vi "test.vi"() -> ()   [LabVIEW 2019]
uses:
  <vilib>/Math Plots/3D Math Plots/3D Surface/3D Surface XCtrl/3D Surface.xctl
  <vilib>/Math Plots/3D Math Plots/3D Surface/3D Surface Datatype/Public/Plot Helper (Vector).vi
  <vilib>/Analysis/NI_AALBase.lvlib
  <vilib>/Math Plots/3D Math Plots/3D Surface/3D Surface Datatype/3D Surface Datatype.lvclass
panel:
  out "appended array":u32[][](array[numeric])
  out "output array":i32[][](array[numeric])
  out "CZT Count Map":refnum<class "3D Plot Datatype.lvclass">[](xcontrol)
  out "Histogram Graph":T1(graph)
  out "Channel":u32[](array[numeric])
  out "Energy":u32[](array[numeric])
  out "Chan+Energy":u32[](array[numeric]) format="%.0x"
  out "Clk Ticks":u32[](array[numeric])
  out "Sr No":i32[](array[numeric])
  # "Sr. No."
  # "Clk Tick"
  # "Raw Data"
  # "Channel"
  # "Energy"
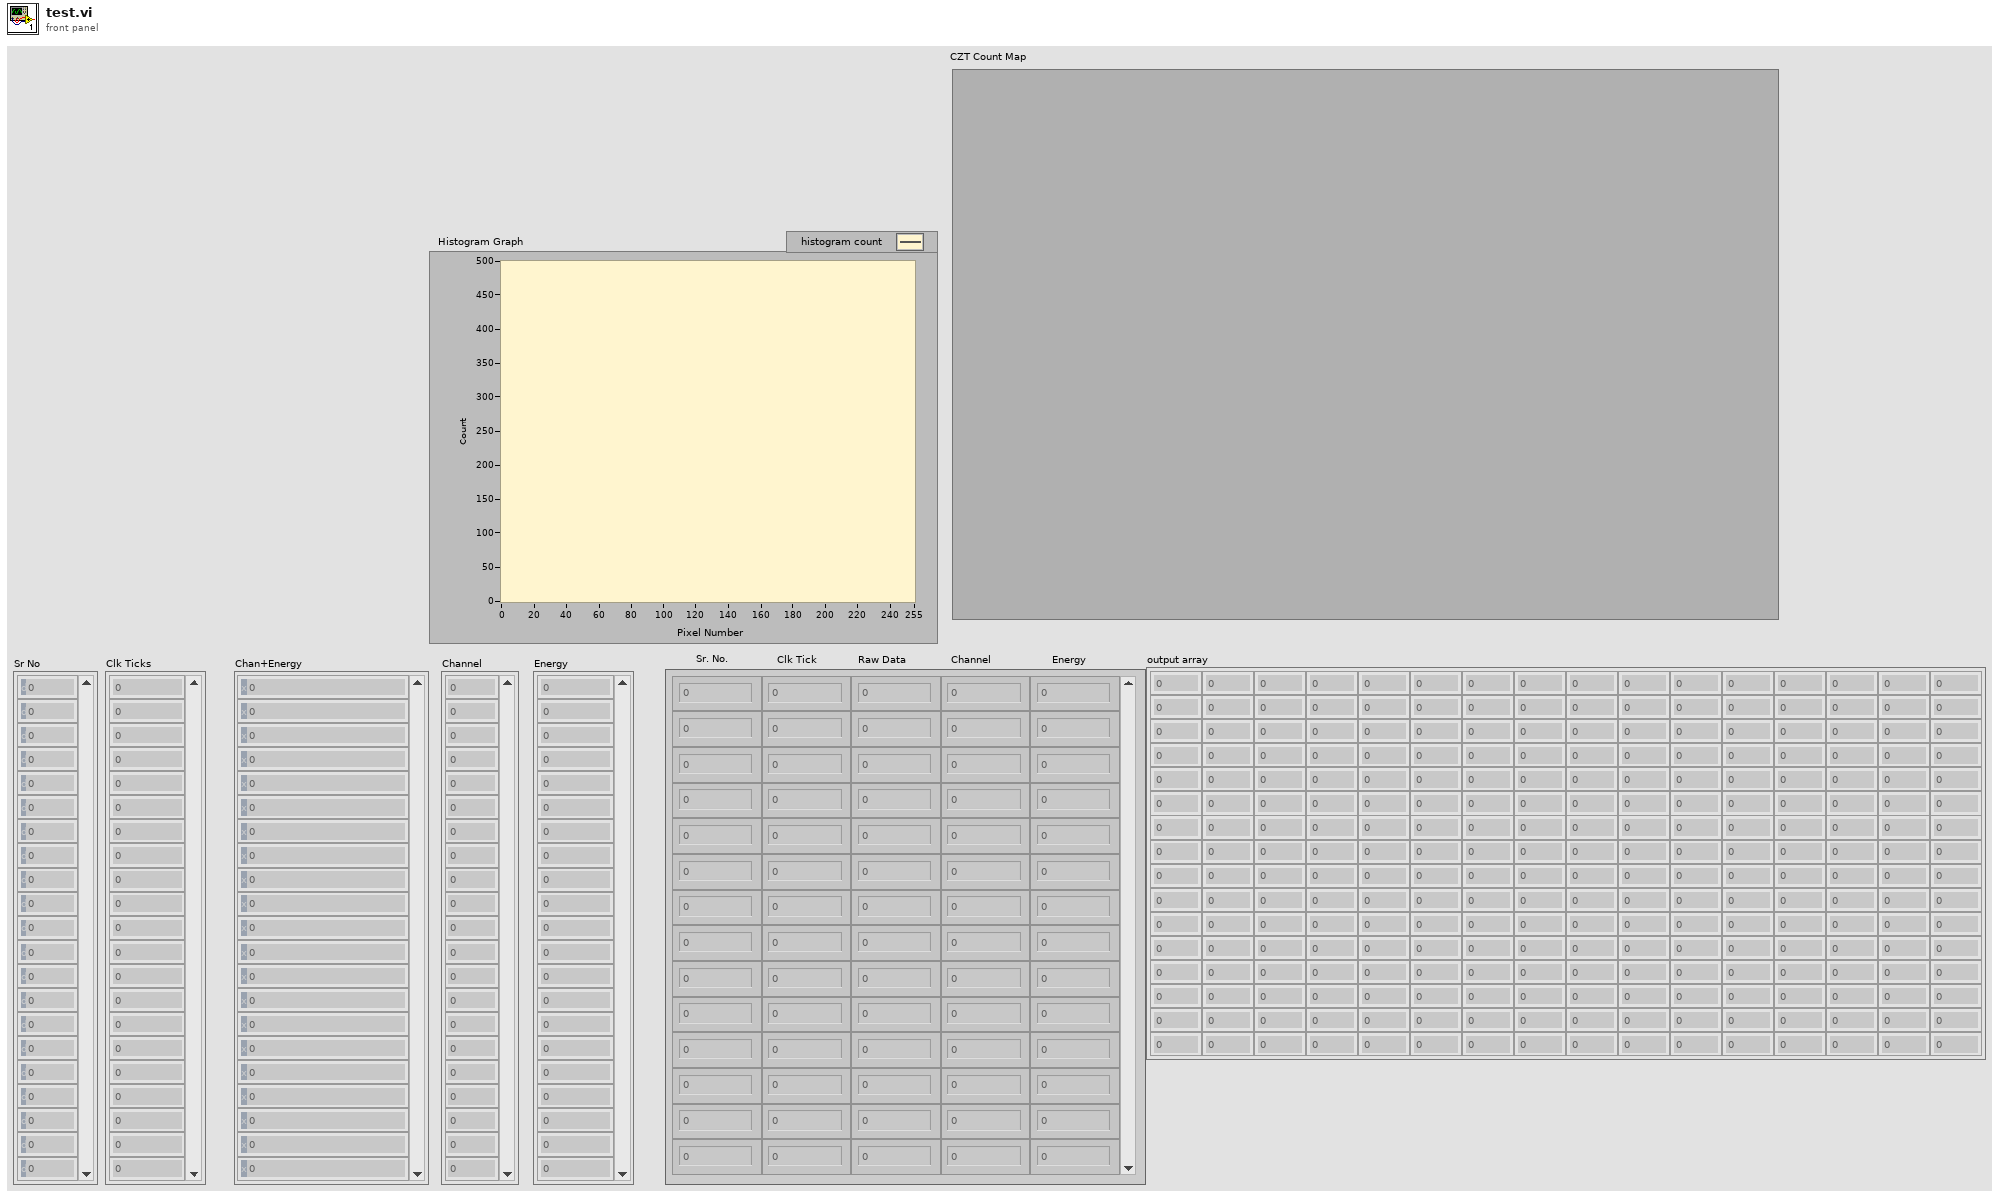
[diagram p1: front panel]
types:
  T1 = cluster{"X Values":dbl[], "Histogram: h(x)":i32[]}
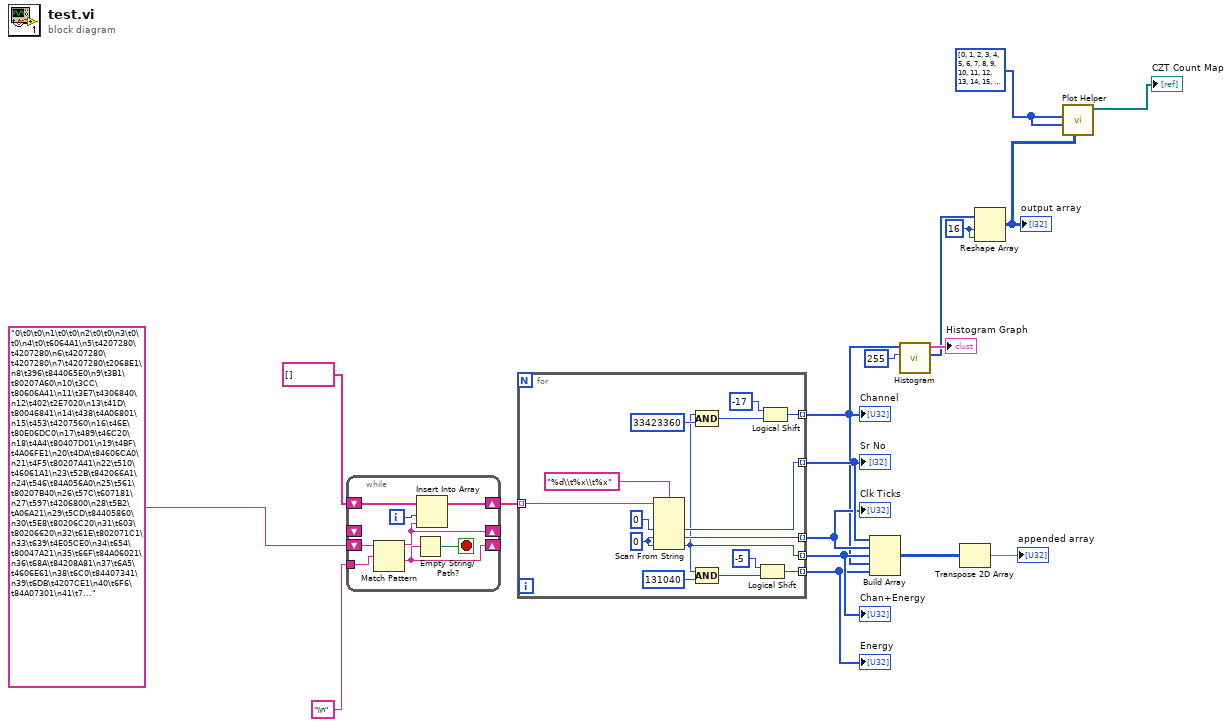
[diagram p0: block diagram]
diagram:
  w1 = u8[] [0, 1, 2, 3, 4, 5, 6, 7, 8, 9, 10, 11, 12, 13, 14, 15, 0, 1, 2, 3, 4, 5, 6, 7, 8, 9, 10, 11, 12, 13, 14, 15, 0, 1, 2, 3, 4, 5, 6, 7, 8, 9, 10, 11, 12, 13, 14, 15, 0, 1, 2, 3, 4, 5, 6, 7, 8, 9, 10, 11, 12, 13, 14, 15, 0, 1, 2, 3, 4, 5, 6, 7, 8, 9, 10, 11, 12, 13, 14, 15, 0, 1, 2, 3, 4, 5, 6, 7, 8, 9, 10, 11, 12, 13, 14, 15, 0, 1, 2, 3, 4, 5, 6, 7, 8, 9, 10, 11, 12, 13, 14, 15, 0, 1, 2, 3, 4, 5, 6, 7, 8, 9, 10, 11, 12, 13, 14, 15, 0, 1, 2, 3, 4, 5, 6, 7, 8, 9, 10, 11, 12, 13, 14, 15, 0, 1, 2, 3, 4, 5, 6, 7, 8, 9, 10, 11, 12, 13, 14, 15, 0, 1, 2, 3, 4, 5, 6, 7, 8, 9, 10, 11, 12, 13, 14, 15, 0, 1, 2, 3, 4, 5, 6, 7, 8, 9, 10, 11, 12, 13, 14, 15, 0, 1, 2, 3, 4, 5, 6, 7, 8, 9, 10, 11, 12, 13, 14, 15, 0, 1, 2, 3, 4, 5, 6, 7, 8, 9, 10, 11, 12, 13, 14, 15, 0, 1, 2, 3, 4, 5, 6, 7, 8, 9, 10, 11, 12, 13, 14, 15, 0, 1, 2, 3, 4, 5, 6, 7, 8, 9, 10, 11, 12, 13, 14] ("Array")
  w4 = 16
  n1 = while {
    tunnel: "\\n" ("regular expression") -> [w25]
    shift-right: [w23] -> _
    shift-left: _ -> [_]
    shift-right: [w20] -> _
    shift-left: "0\t0\t0\n1\t0\t0\n2\t0\t0\n3\t0\t0\n4\t0\t6064A1\n5\t4207280\t4207280\n6\t4207280\t4207280\n7\t4207280\t2068E1\n8\t396\t844065E0\n9\t3B1\t80207A60\n10\t3CC\t80606A41\n11\t3E7\t4306840\n12\t402\t2E7020\n13\t41D\t80046841\n14\t438\t4A06801\n15\t453\t4207560\n16\t46E\t80E06DC0\n17\t489\t46C20\n18\t4A4\t80407D01\n19\t4BF\t4A06FE1\n20\t4DA\t84606CA0\n21\t4F5\t80207A41\n22\t510\t46061A1\n23\t52B\t842066A1\n24\t546\t84A056A0\n25\t561\t80207B40\n26\t57C\t607181\n27\t597\t4206800\n28\t5B2\tA06A21\n29\t5CD\t84405860\n30\t5E8\t80206C20\n31\t603\t80206620\n32\t61E\t802071C1\n33\t639\t4E05CE0\n34\t654\t80047A21\n35\t66F\t84A06021\n36\t68A\t84208A81\n37\t6A5\t4606E61\n38\t6C0\t84407341\n39\t6DB\t4207CE1\n40\t6F6\t84A07301\n41\t711\t4606C60\n42\t72C\t80406D00\n43\t747\t207EE0\n44\t762\t802070A0\n45\t77D\t80406620\n46\t798\t80208AC0\n47\t7B3\t607481\n48\t7CE\t4208900\n49\t7E9\t3871C1\n50\t804\t42E7E21\n51\t81F\t85706541\n52\t83A\t4E06A61\n53\t855\t84506DE0\n54\t870\t80047AA0\n55\t88B\t80307601\n56\t8A6\t4A07C80\n57\t8C1\t20A361\n58\t8DC\t844084E0\n59\t8F7\t80206C80\n60\t912\t6083A1\n61\t92D\t842071A1\n62\t948\t844078A1\n63\t963\t84606AA0\n64\t97E\t80206160\n65\t999\t80206E21\n66\t9B4\t84E05D00\n67\t9CF\t470A0\n68\t9EA\t80A06921\n69\tA05\t84208021\n70\tA20\t84407840\n71\tA3B\t606CE1\n72\tA56\t842067A0\n73\tA71\t80206F40\n74\tA8C\t2075E1\n75\tAA7\t84206920\n76\tAC2\t80206B81\n77\tADD\t44074C1\n78\tAF8\t4047840\n79\tB13\t1846AC1\n80\tB2E\t46061E0\n81\tB49\t80208321\n82\tB64\t84406E60\n83\tB7F\t80206F01\n84\tB9A\t4206920\n85\tBB5\t80206661\n86\tBD0\t84207A60\n87\tBEB\t80608040\n88\tC06\t208381\n89\tC21\t4406B00\n90\tC3C\t206DA0\n91\tC57\t80206860\n92\tC72\t80206A80\n93\tC8D\t206CE0\n94\tCA8\t80206141\n95\tCC3\t4406561\n96\tCDE\t84207D61\n97\tCF9\t84207CE1\n98\tD14\t84306D61\n99\tD2F\t84E065C1\n100\tD4A\t4047120\n101\tD65\t80A067C1\n102\tD80\t4208D80\n103\tD9B\t607D00\n104\tDB6\t408220\n105\tDD1\t80208E01\n106\tDEC\t4605E80\n107\tE07\t406AA1\n108\tE22\t842071A1\n109\tE3D\t84207660\n110\tE58\t80206BE1\n111\tE73\t842061C0\n112\tE8E\t206540\n113\tEA9\t206EA0\n114\tEC4\t80206181\n115\tEDF\t42069C1\n116\tEFA\t4406F20\n117\tF15\t80207240\n118\tF30\t207021\n119\tF4B\t84406400\n120\tF66\t208321\n121\tF81\t84207880\n122\tF9C\t2077A1\n123\tFB7\t84206C40\n124\tFD2\t605EE0\n125\tFED\t800468E1\n126\t1008\t84406B81\n127\t1023\t42090A1\n128\t103E\t842072C1\n129\t1059\t4FC5921\n130\t1074\t85AE7421\n131\t108F\t84F073C1\n132\t10AA\t5C268E0\n133\t10C5\t80387021\n134\t10E0\t850E6C21\n135\t10FB\t84327E61\n136\t1116\t84E08EA1\n137\t1131\t859075C0\n138\t114C\t12E5620\n139\t1167\t80D07581\n140\t1182\t4048861\n141\t119D\t85507041\n142\t11B8\t42E83A1\n143\t11D3\t84707060\n144\t11EE\t80A08F61\n145\t1209\t85706081\n146\t1224\t44E6EA1\n147\t123F\t84B06181\n148\t125A\t420B981\n149\t1275\t4307A61\n150\t1290\t848E70E0\n151\t12AB\t80906F00\n152\t12C6\t6092A1\n153\t12E1\t84365F00\n154\t12FC\t409061\n155\t1317\t84507F61\n156\t1332\t84206301\n157\t134D\t4205A01\n158\t1368\t4A05220\n159\t1383\t80046700\n160\t139E\t607A20\n161\t13B9\t80207740\n162\t13D4\t4077C1\n163\t13EF\t40458E1\n164\t140A\t84606CE1\n165\t1425\t84208440\n166\t1440\t4065E0\n167\t145B\t80305480\n168\t1476\t2E8520\n169\t1491\t80366740\n170\t14AC\t47BC1\n171\t14C7\t4507CA1\n172\t14E2\t84E07000\n173\t14FD\t20A680\n174\t1518\tA08200\n175\t1533\t607841\n176\t154E\t4409160\n177\t1569\t80205B41\n178\t1584\t4205F20\n179\t159F\t81DC52C1\n180\t15BA\t58E7500\n181\t15D5\t1D275A0\n182\t15F0\t81C66340\n183\t160B\t5C7E60\n184\t1626\t80EE66C0\n185\t1641\t3479A0\n186\t165C\t80E090E0\n187\t1677\t81DC5740\n188\t1692\t16E9321\n189\t16AD\t85307201\n190\t16C8\t5A46921\n191\t16E3\t84388681\n192\t16FE\t42C64E1\n193\t1719\t84D08D80\n194\t1734\t4A2A0\n195\t174F\t81D85EE1\n196\t176A\t85AE9381\n197\t1785\t5D084A0\n198\t17A0\t81C66940\n199\t17BB\t7A72E0\n200\t17D6\t806E6061\n201\t17F1\t84327F00\n202\t180C\tA08C40\n203\t1827\t1DA60E1\n204\t1842\t852E6BE1\n205\t185D\t85B07FC1\n206\t1878\t5C47A61\n207\t1893\t84388261\n208\t18AE\t84286261\n209\t18C9\t843085E0\n210\t18E4\t8020AE21\n211\t18FF\t85DC8001\n212\t191A\t58E7720\n213\t1935\t81D467A0\n214\t1950\t81C290C0\n215\t196B\tBA6601\n216\t1986\t4CE64C0\n217\t19A1\t347A21\n218\t19BC\t84E09A80\n219\t19D7\t5A7121\n220\t19F2\t854E77C1\n221\t1A0D\t51070A1\n222\t1A28\t85A26E01\n223\t1A43\t43A6681\n224\t1A5E\t42C6561\n225\t1A79\t84B06E00\n226\t1A94\t48DA1\n227\t1AAF\t84FC7DE1\n228\t1ACA\t85AE7121\n229\t1AE5\t85D068C1\n230\t1B00\t4327560\n231\t1B1B\t810E6840\n232\t1B36\t3CB200\n233\t1B51\tE079A0\n234\t1B6C\t81D08B60\n235\t1B87\t816E7760\n236\t1BA2\t803C9560\n237\t1BBD\t81C273C1\n238\t1BD8\t4B069A1\n239\t1BF3\t842E6E40\n240\t1C0E\t3C91C1\n241\t1C29\t40460A1\n242\t1C44\t85306E00\n243\t1C5F\t1C860C0\n244\t1C7A\t3CACC0\n245\t1C95\tA07961\n246\t1CB0\t847067E1\n247\t1CCB\t852E6D81\n248\t1CE6\t43C9660\n249\t1D01\t80207900\n250\t1D1C\t1D08700\n251\t1D37\t1AE6E80\n252\t1D52\t3CEDC0\n253\t1D6D\tE07120\n254\t1D88\t80D07000\n255\t1DA3\t12E6920\n256\t1DBE\t803CE760\n257\t1DD9\t80045E00\n258\t1DF4\t19083C0\n259\t1E0F\t406721\n260\t1E2A\t843CB4A0\n261\t1E45\t802089E1\n262\t1E60\t84307181\n263\t1E7B\t4A07C40\n264\t1E96\t3C7501\n265\t1EB1\t42E7AE0\n266\t1ECC\t81D06A21\n267\t1EE7\t84044D01\n268\t1F02\t43CBCA1\n269\t1F1D\t858E6B41\n270\t1F38\t4326D41\n271\t1F53\t4E08EC1\n272\t1F6E\t43C76E0\n273\t1F89\t80209281\n274\t1FA4\t4967601\n275\t1FBF\t48E7460\n276\t1FDA\t80987621\n277\t1FF5\t85C67B01\n278\t2010\t4907301\n279\t202B\t54E82A1\n280\t2046\t851C60E1\n281\t2061\t84606DE0\n282\t207C\t81D480E1\n283\t2097\t842C7861\n284\t20B2\t855C7461\n285\t20CD\t85626F60\n286\t20E8\t80526F20\n287\t2103\t81C88C20\n288\t211E\t80DC6200\n289\t2139\t247221\n290\t2154\t855079C0\n291\t216F\tCE7C41\n292\t218A\t53C7A21\n293\t21A5\t85C46621\n294\t21C0\t843662C1\n295\t21DB\t52E7BC1\n296\t21F6\t4386B21\n297\t2211\t84E0C100\n298\t222C\t1526381\n299\t2247\t4286FA0\n300\t2262\t81BC6B20\n301\t227D\t81847A81\n302\t2298\t4347C21\n303\t22B3\t858E9C61\n304\t22CE\t847C6C01\n305\t22E9\t42677C1\n306\t2304\t5306F61\n307\t231F\t846E73E1\n308\t233A\t84787460\n309\t2355\t81C27340\n310\t2370\tD098A0\n311\t238B\t816E7F80\n312\t23A6\t386721\n313\t23C1\t84A08A80\n314\t23DC\t1D27401\n315\t23F7\t42A61E1\n316\t2412\t85D87E20\n317\t242D\t81026401\n318\t2448\t432A1A0\n319\t2463\t81AE9120\n320\t247E\t80BC6F80\n321\t2499\t4A340\n322\t24B4\t1B07121\n323\t24CF\t84EE7A61\n324\t24EA\t85DCA740\n325\t2505\t1C25960\n326\t2520\t80307CE0\n327\t253B\t818E6121\n328\t2556\t84386C61\n329\t2571\t84E086C0\n330\t258C\t1D67481\n331\t25A7\t42E93C0\n332\t25C2\t17C7400\n333\t25DD\t1A45B80\n334\t25F8\tB08B61\n335\t2613\t84AE7621\n336\t262E\t843C7F80\n337\t2649\t2087E0\n338\t2664\t80B65DA0\n339\t267F\t810E82C0\n340\t269A\t1DA8100\n341\t26B5\t4075E1\n342\t26D0\t84707D20\n343\t26EB\t804E7E41\n344\t2706\t49C7281\n345\t2721\t4047560\n346\t273C\t81926AC0\n347\t2757\tA08841\n348\t2772\t43A7241\n349\t278D\t4207161\n350\t27A8\t849084E1\n351\t27C3\t84E06580\n352\t27DE\t5A8741\n353\t27F9\t4047761\n354\t2814\t857063C0\n355\t282F\t607721\n356\t284A\t843C76C1\n357\t2865\t5AE7421\n358\t2880\t84327300\n359\t289B\t1C26861\n360\t28B6\t85DC65E1\n361\t28D1\t842E8080\n362\t28EC\t1D07E00\n363\t2907\t20BAC0\n364\t2922\t7A76E1\n365\t293D\t858E6160\n366\t2958\t80307A20\n367\t2973\t80E086C0\n368\t298E\t5C7CA1\n369\t29A9\t850E6A21\n370\t29C4\t851069E1\n371\t29DF\t840497E1\n372\t29FA\t84FC7221\n373\t2A15\t84A06D80\n374\t2A30\tD07560\n375\t2A4B\t80205FA1\n376\t2A66\t843C74A0\n377\t2A81\t80E06D41\n378\t2A9C\t5D07481\n379\t2AB7\t56E7020\n380\t2AD2\t81DC6280\n381\t2AED\t1C26E80\n382\t2B08\t327DC1\n383\t2B23\t42E72A0\n384\t2B3E\t80387EA1\n385\t2B59\t840491E1\n386\t2B74\t85907BE0\n387\t2B8F\t81AE7B00\n388\t2BAA\tFC5FC0\n389\t2BC5\t406A80\n390\t2BE0\t508040\n391\t2BFB\t4E5840\n392\t2C16\t3C88E1\n393\t2C31\t8420A320\n394\t2C4C\t80F07E21\n395\t2C67\t858E7360\n396\t2C82\t80B05F01\n397\t2C9D\t4E08180\n398\t2CB8\t15070A0\n399\t2CD3\t80CE6020\n400\t2CEE\t80309581\n401\t2D09\t4206FC1\n402\t2D24\t5B06D40\n403\t2D3F\tA08FC1\n404\t2D5A\t4905DC1\n405\t2D75\t46096C0\n406\t2D90\t1707181\n407\t2DAB\t44061A0\n408\t2DC6\t80707F41\n409\t2DE1\t4046580\n410\t2DFC\t306C60\n411\t2E17\t80E070A0\n412\t2E32\t80208261\n413\t2E4D\t84A07F20\n414\t2E68\t80206221\n415\t2E83\t84607400\n416\t2E9E\t407740\n417\t2EB9\t2063C1\n418\t2ED4\t4205E00\n419\t2EEF\t1D05A21\n420\t2F0A\t85AE7901\n421\t2F25\t4327220\n422\t2F40\t80E07000\n423\t2F5B\tF07361\n424\t2F76\t842E6701\n425\t2F91\t4386DA0\n426\t2FAC\t81C27A20\n427\t2FC7\t80365D01\n428\t2FE2\t58E6BA0\n429\t2FFD\t81D069E1\n430\t3018\t84047DE0\n431\t3033\t80328120\n432\t304E\t802E6820\n433\t3069\t81B06E61\n434\t3084\t84A087A0\n435\t309F\t80306060\n436\t30BA\t81AE75E0\n437\t30D5\t80707740\n438\t30F0\t208AC0\n439\t310B\t507C01\n440\t3126\t4E07581\n441\t3141\t4608FE0\n442\t315C\t80408AC0\n443\t3177\t205D21\n444\t3192\t84205AC1\n445\t31AD\t4605B01\n446\t31C8\t4047461\n447\t31E3\t84406920\n448\t31FE\t802080A0\n449\t3219\t80205E00\n450\t3234\tA05FC0\n451\t324F\t471C1\n452\t326A\t4607400\n453\t3285\t2076A0\n454\t32A0\t804071E0\n455\t32BB\t802070E1\n456\t32D6\t85D85D21\n457\t32F1\t848E7DC0\n458\t330C\t1D474C1\n459\t3327\t5C66141\n460\t3342\t45A7340\n461\t335D\t12E6680\n462\t3378\t328341\n463\t3393\t4E09160\n464\t33AE\t81DA62A1\n465\t33C9\t842C6E00\n466\t33E4\t1306061\n467\t33FF\t1A46541\n468\t341E\t388E40\n469\t3451\t18E6C01\n470\t3482\tD08541\n471\t34B5\t493E0\n472\t34E6\t1DC6341\n473\t3519\tEE7160\n474\t354A\t1D07800\n475\t357D\t1C265E1\n476\t35AE\t3C7FC1\n477\t35E1\t14E5B00\n478\t3612\t3085E0\n479\t3645\tA09120\n480\t3676\tFC67E0\n481\t36A9\t2E8B60\n482\t36DA\t15063E0\n483\t370D\t20B401\n484\t373E\tB06881\n485\t3771\t1AE6E20\n486\t37A2\t1D879A0\n487\t37D5\t1C65D81\n488\t3806\t1D26800\n489\t3839\t6E7581\n490\t386A\t3863E0\n491\t389D\tE06E60\n492\t38CE\t327401\n493\t3901\t16E6660\n494\t3932\t1DC7601\n495\t3965\t1A46101\n496\t3996\t1107361\n497\t39C9\t2E85A1\n498\t39FA\t3C6820\n499\t3A2D\t46821\n500\t3A5E\t707FC0\n501\t3A91\t18E6F20\n502\t3AC2\t1DC7FC1\n503\t3AF5\t1C45D80\n504\t3B26\t1D08121\n505\t3B59\tCE6F80\n506\t3B8A\t325FC1\n507\t3BBD\t60A600\n508\t3BEE\t19067A0\n509\t3C21\t1AE7721\n510\t3C52\tD07A21\n511\t3C85\t1C26000\n512\t3CB6\t3877C1\n513\t3CE9\t2E8301\n514\t3D1A\t1D26400\n515\t3D4D\t207021\n516\t3D7E\t1DC6A81\n517\t3DB1\t12E6BC0\n518\t3DE2\t326F61\n519\t3E15\tE081A1\n520\t3E46\t3A6E80\n521\t3E79\tAE62E1\n522\t3EAA\t13067C0\n523\t3EDD\t46D21\n524\t3F0E\t385241\n525\t3F41\t18E7921\n526\t3F72\t308281\n527\t3FA5\t1C27241\n528\t3FD6\t3C8E21\n529\t4009\t2E74A0\n530\t403A\t1D06AE1\n531\t406D\tA07C20\n532\t409E\t327941\n533\t40D1\t16E7301\n534\t4102\t1D85EA0\n535\t4135\t1C475E0\n536\t4166\t1706EA1\n537\t4199\t10E60C0\n538\t41CA\t388780\n539\t41FD\t208681\n540\t422E\t906880\n541\t4261\t1C88561\n542\t4292\t1BC6220\n543\t42C5\t1C67761\n544\t42F6\t1B26F20\n545\t4329\t2A6821\n546\t435A\tBC6640\n547\t438D\tE08041\n548\t43BE\t526421\n549\t43F1\tEC6F20\n550\t4422\t17C6DC1\n551\t4455\t1426FE0\n552\t4486\tF07800\n553\t44B9\t4E7721\n554\t44EA\t11C73E0\n555\t451D\t48321\n556\t454E\t367760\n557\t4581\t18E67C0\n558\t45B2\t1DC75C1\n559\t45E5\t1C27B60\n560\t4616\t1D66120\n561\t4649\t287AC1\n562\t467A\t7C6AC1\n563\t46AD\t409601\n564\t46DE\t3482A1\n565\t4711\t14E65C1\n566\t4742\t1D881E0\n567\t4775\t1026861\n568\t47A6\t1B06CE1\n569\t47D9\tCE7BA1\n570\t480A\t3872C1\n571\t483D\t206400\n572\t486E\tD07A41\n573\t48A1\t1AE52A1\n574\t48D2\t1DA8741\n575\t4905\t1825E60\n576\t4936\t1D45C61\n577\t4969\t2C78E0\n578\t499A\t5A6FE1\n579\t49CD\tA066A0\n580\t49FE\t327801\n581\t4A31\t12E8801\n582\t4A62\t3C6740\n583\t4A95\t1A46921\n584\t4AC6\t1307861\n585\t4AF9\t8E7421\n586\t4B2A\tFC72E1\n587\t4B5D\t207420\n588\t4B8E\t306780\n589\t4BC1\t16E6960\n590\t4BF2\t5C84E1\n591\t4C25\t1A26000\n592\t4C56\t1D06C00\n593\t4C89\t2E6B61\n594\t4CBA\t3A7700\n595\t4CED\tE06B81\n596\t4D1E\tB06700\n597\t4D51\tEE6DE0\n598\t4D82\t1506680\n599\t4DB5\t1C46381\n600\t4DE6\t7082C1\n601\t4E19\t6E6DE1\n602\t4E4A\t1D27EC1\n603\t4E7D\t2081A1\n604\t4EAE\t507AE0\n605\t4EE1\t10E9060\n606\t4F12\t1106581\n607\t4F45\t608AE0\n608\t4F76\t1907161\n609\t4FA9\tAE6DA0\n610\t4FDA\t1708080\n611\t500D\t207A60\n612\t503E\t405E41\n613\t5071\t606EE0\n614\t50A2\t206AA1\n615\t50EF\t607061\n616\t5120\t205F40\n617\t5E99\t206441\n618\t835E\t206B00\n619\t88DB\t205580\n620\t8AAC\tE05940\n621\t93B7\t2091A0\n622\t93E8\tA06E40\n623\t941B\t406AC1\n624\t944C\t6072A0\n625\t947F\t206580\n626\tB314\t206540\n627\tB457\t205E81\n628\tB80E\t2063C1\n629\tD0F7\t207261\n630\tE6C2\t606941\n631\tE7ED\t206BE1\n632\tE81E\t206C61\n633\tEDC1\t207681\n634\tEF78\t2066E0\n635\tF0A3\t207300\n636\tF5EA\t207521\n637\tF679\t2073C0\n638\tF88C\t206421\n639\tF969\t2073E1\n640\tF9F6\t606900\n641\tFB6F\t2070E1\n642\tFBA0\t606EA1\n643\tFBD3\t2073A0\n644\tFC04\t206E00\n645\tFD77\t206DE1\n646\tFEA2\t206EA0\n647\tFEEF\t206EA0\n648\tFF3E\tA05D40\n649\tFFCD\t476E1\n650\tFFFE\t407360\n651\t10031\t2083C0\n652\t10062\t606F60\n653\t10095\t205CE0\n654\t10134\tD06181\n655\t103E9\t2E71A0\n656\t1041A\t3072C0\n657\t1044D\tE06A61\n658\t1047E\t506140\n659\t104B1\t47D61\n660\t104E2\tA077E1\n661\t10515\t20A361\n662\t10546\t407A21\n663\t10579\t6078E1\n664\t105AA\t206920\n665\t10769\t4070C0\n666\t107F6\t47081\n667\t10829\t607741\n668\t1085A\t208880\n669\t1088D\t206160\n670\t108E0\t208000\n671\t10923\t2066C1\n672\t10D3C\tD06C01\n673\t110BD\t2E6B20\n674\t110EE\tE06DC0\n675\t11121\t46E81\n676\t11152\tA06180\n677\t11185\t2082E0\n678\t111B6\t406901\n679\t111E9\t606DA1\n680\t1121A\t206080\n681\t1126F\t208720\n682\t11432\t207140\n683\t11721\t4074C1\n684\t117B2\t208041\n685\t117E5\t606F21\n686\t11816\t326F20\n687\t11977\t2E7400\n688\t119A8\t7A6FE0\n689\t119DB\t1C263A0\n690\t11A0C\t3074E1\n691\t11A3F\t48A60\n692\t11A70\tD07280\n693\t11AA3\tE08240\n694\t11AD4\t706F20\n695\t11B07\t20AB00\n696\t11B38\t5071A0\n697\t11B6B\tA08020\n698\t11B9C\t409700\n699\t11BCF\t608301\n700\t11C00\t1D863A1\n701\t11CF7\t12E70E1\n702\t11D28\t13068A0\n703\t11D5B\t1C65AA1\n704\t11D8C\t387000\n705\t11DBF\tCE6940\n706\t11DF0\t327AC0\n707\t11E23\t49CE0\n708\t11E54\t1506C20\n709\t11E87\t16E5140\n710\t11EB8\t906F00\n711\t11EEB\t1A46321\n712\t11F1C\tF08141\n713\t11F4F\t2A5C40\n714\t11F80\t307F40\n715\t11FB3\tE08880\n716\t11FE4\t1706E20\n717\t12017\t4E6F00\n718\t12048\tD07C81\n719\t1207B\t1C26EA1\n720\t120AC\t1107400\n721\t120DF\t2E7A20\n722\t12110\t707F00\n723\t12143\t20AC61\n724\t12174\t366E20\n725\t121A7\tEE6541\n726\t121D8\t508340\n727\t1220B\tA08F20\n728\t1223C\t3072C0\n729\t1226F\t2E71A0\n730\t122A0\t5068A1\n731\t122D3\t485C0\n732\t12304\t8E6E80\n733\t12337\tE08140\n734\t12368\t10E74E1\n735\t1239B\t20A6E0\n736\t123CC\t6E61E1\n737\t123FF\t4091C0\n738\t12430\t609880\n739\t12463\t5A5F00\n740\t125BC\t16E7620\n741\t125EF\t1906821\n742\t12620\t1C27141\n743\t12653\t386D60\n744\t12684\t2E85A1\n745\t126B7\t327CA0\n746\t126E8\t49860\n747\t1271B\tFC6E80\n748\t1274C\tEE4B81\n749\t1277F\t1106CA0\n750\t127B0\tE08360\n751\t127E3\t908020\n752\t12814\t4E7301\n753\t12847\t1506BE1\n754\t12878\t20AB41\n755\t128AB\t308200\n756\t128DC\t10E6B20\n757\t1290F\t17066C0\n758\t12940\tA080C1\n759\t12973\t707480\n760\t129A4\t206821\n761\t129D7\t3673A1\n762\t12A08\t409020\n763\t12A3B\t507E21\n764\t12A6C\t6086A1\n765\t12A9F\t47840\n766\t12AF4\t1846B60\n767\t12B27\tE07120\n768\t12B58\t208581\n769\t12B8B\tA06401\n770\t12BBC\t407DE0\n771\t12BEF\t607200\n772\t12C20\t206E81\n773\t12D4B\t405AC1\n774\t12E74\tF06A81\n775\t12EA7\t470C0\n776\t12ED8\t326361\n777\t12F0B\tE06760\n778\t12F3C\tD07500\n779\t12F6F\t207C21\n780\t12FA0\t306BC1\n781\t12FD3\tA06F81\n782\t13004\t365880\n783\t13037\t206E21\n784\t13068\t506E20\n785\t1309B\tE070C0\n786\t130CC\t6072A0\n787\t130FF\tA060A0\n788\t13130\t405881\n789\t13163\t46781\n790\t133BA\t3276E1\n791\t133ED\t2E6840\n792\t1341E\t906621\n793\t13451\t1846481\n794\t13482\t308580\n795\t134B5\t4E6AE1\n796\t134E6\t366D40\n797\t13519\tE061E1\n798\t1354A\t506440\n799\t1357D\t2E6581\n800\t135AE\t3A6D01\n801\t135E1\t20AAA1\n802\t13612\t306C60\n803\t13645\tA05EA1\n804\t13676\t472E0\n805\t136A9\tE07521\n806\t136DA\t2073A0\n807\t1370D\t607CC1\n808\t1373E\t463E0\n809\t13771\tE068A0\n810\t137A2\t207C81\n811\t137D5\tA06C00\n812\t13806\t477A1\n813\t13839\tE070C0\n814\t1386A\t4069A1\n815\t1389D\t607141\n816\t138CE\t206841\n817\t13901\t406F01\n818\t13932\t205F20\n819\t1398F\t605440\n820\t13AE0\t207401\n821\t13B13\t207740\n822\t13C9E\t2071A1\n823\t13D0F\tF06621\n824\t13E3A\t2E73C1\n825\t13E6D\tD062A0\n826\t13E9E\tE067E1\n827\t13ED1\t506521\n828\t13F02\t47240\n829\t13F35\t307241\n830\t13F66\tA076C1\n831\t13F99\t2092A0\n832\t13FCA\t4084C1\n833\t13FFD\t13C6EA0\n834\t1402E\t1AE8E41\n835\t14061\t1526C41\n836\t14092\t1C673A0\n837\t140C5\t11C6B80\n838\t140F6\tCE6CC1\n839\t14129\tD47460\n840\t1415A\t426EA1\n841\t1418D\t19C7300\n842\t141BE\t12E6601\n843\t141F1\t1B66F41\n844\t14222\t1826961\n845\t14255\tDC7381\n846\t14286\t2C7641\n847\t142B9\tB07401\n848\t142EA\tE09501\n849\t1431D\t17C7181\n850\t1434E\t14E6281\n851\t14381\t1308480\n852\t143B2\t1225F01\n853\t143E5\t387E40\n854\t14416\tAE7600\n855\t14449\t328960\n856\t1447A\t266961\n857\t144AD\t1BC7380\n858\t144DE\t16E84C0\n859\t14511\t15076E1\n860\t14542\t1C28920\n861\t14575\t7C7021\n862\t145A6\t2866C0\n863\t145D9\t708E20\n864\t1460A\tA0A2E0\n865\t1463D\t1D87BA1\n866\t1466E\tEE7B81\n867\t146A1\t966F21\n868\t146D2\t1026D20\n869\t14705\tBC71A1\n870\t14736\t2A6421\n871\t14769\t5274A1\n872\t1479A\t49E81\n873\t147CD\t1DA7C20\n874\t147FE\t6E79E1\n875\t14831\t1907840\n876\t14862\t1A27361\n877\t14895\t5C77C0\n878\t148C6\t2E9480\n879\t148F9\tD071A1\n880\t1492A\tE05980\n881\t1495D\t9C6660\n882\t1498E\t10E7501\n883\t149C1\tF082C0\n884\t149F2\t1A47221\n885\t14A25\t3A68A1\n886\t14A56\t8E7721\n887\t14A89\t3095C0\n888\t14ABA\t20C441\n889\t14AED\t5A7B00\n890\t14B1E\t4E76C1\n891\t14B51\t1708200\n892\t14B82\t1C46CA0\n893\t14BB5\tFC7700\n894\t14BE6\t606D01\n895\t14C19\t908601\n896\t14C4A\t47861\n897\t14C7D\t11084E1\n898\t14CAE\tE06A01\n899\t14CE1\t368121\n900\t14D12\t209EE1\n901\t14D45\t1B07020\n902\t14D76\tA06861\n903\t14DA9\t306E01\n904\t14DDA\t40B560\n905\t14E0D\t5094E0\n906\t14E3E\t607A01\n907\t14E71\t206E00\n908\t14EA2\t4063A1\n909\t14ED5\t6076A1\n910\t14F06\t2076C0\n911\t14FB7\t4056E0\n912\t17346\t207541\n913\t17379\t2051C0\n914\t17760\t206800\n915\t178DD\t205EA0\n916\t1792C\t305621\n917\t1AED9\tE05860\n918\t1AF0A\t5051E0\n919\t1AF3D\t47DA1\n920\t1AF6E\tA07100\n921\t1AFA1\t208FC0\n922\t1AFD2\t607F61\n923\t1B005\t18E5640\n924\t1B036\t1DC4E41\n925\t1B069\t1C666C1\n926\t1B09A\t1D455A1\n927\t1B0CD\t2C7401\n928\t1B0FE\t11C6F21\n929\t1B131\t46D00\n930\t1B162\tB26E80\n931\t1B195\t12E4C60\n932\t1B1C6\t13C65E0\n933\t1B1F9\t12262C0\n934\t1B22A\t1305D00\n935\t1B25D\tCE7960\n936\t1B28E\t5C64E0\n937\t1B2C1\tE090A1\n938\t1B2F2\tD0A400\n939\t1B325\t14C71E1\n940\t1B356\t15C9680\n941\t1B389\t1467040\n942\t1B3BA\t1D66A41\n943\t1B3ED\tAC8361\n944\t1B41E\tD88400\n945\t1B451\tA27F41\n946\t1B482\t348B01\n947\t1B4B5\t10A7581\n948\t1B4E6\t19887E1\n949\t1B519\t1247740\n950\t1B54A\t1567780\n951\t1B57D\tA87E20\n952\t1B5AE\tFA8920\n953\t1B5E1\tA68001\n954\t1B612\tF48420\n955\t1B645\t12A76C1\n956\t1B676\t1BA8DA0\n957\t1B6A9\tE46A60\n958\t1B6DA\t1B48AE1\n959\t1B70D\t4A77A1\n960\t1B73E\t1186221\n961\t1B771\t4491E0\n962\t1B7A2\t948261\n963\t1B7D5\t12869A1\n964\t1B806\t988C21\n965\t1B839\t1427621\n966\t1B86A\tB69760\n967\t1B89D\t1688460\n968\t1B8CE\tDA7FA0\n969\t1B901\tC65660\n970\t1B932\tD679A0\n971\t1B965\t14A83A1\n972\t1B996\t15A9481\n973\t1B9C9\t1A66E00\n974\t1B9FA\t1948A20\n975\t1BA2D\t2870C1\n976\t1BA5E\t385DA0\n977\t1BA91\t26A100\n978\t1BAC2\t548461\n979\t1BAF5\t1AE78A0\n980\t1BB26\t1587F40\n981\t1BB59\t1445620\n982\t1BB8A\t1969040\n983\t1BBBD\t687AA0\n984\t1BBEE\t7A7AE1\n985\t1BC21\t4688C1\n986\t1BC52\t567441\n987\t1BC85\t18C86A1\n988\t1BCB6\t17A93A0\n989\t1BCE9\t1C65580\n990\t1BD1A\t1D27CA0\n991\t1BD4D\t8A73A0\n992\t1BD7E\t5873C0\n993\t1BDB1\t847D81\n994\t1BDE2\tF26C01\n995\t1BE15\t1887541\n996\t1BE46\t13A7C81\n997\t1BE79\t1647460\n998\t1BEAA\t1347D81\n999\t1BEDD\tCA65E1\n1000\t1BF0E\tBA86C0\n1001\t1BF41\t16671C1\n1002\t1BF72\t1128401\n1003\t1BFA5\t18A8BE1\n1004\t1BFD6\t19A7D20\n1005\t1C009\tE277E1\n1006\t1C03A\t15488A0\n1007\t1C06D\t6C6941\n1008\t1C09E\t11A7C20\n1009\t1C0D1\t647801\n1010\t1C102\t326640\n1011\t1C135\t1087CE0\n1012\t1C166\t1B878A1\n1013\t1C199\t1C27281\n1014\t1C1CA\t1768860\n1015\t1C1FD\t885500\n1016\t1C22E\t9A7760\n1017\t1C261\t866C80\n1018\t1C292\tF67400\n1019\t1C2C5\t1AA8FC0\n1020\t1C2F6\t1BC83E0\n1021\t1C329\t1268080\n1022\t1C35A\t1B29441\n1023\t1C38D\t4C6B60\n1024\t1C3BE\tB88B00\n1025\t1C3F1\t247B00\n1026\t1C422\t927C00\n1027\t1C455\tEA7801\n1028\t1C486\t788481\n1029\t1C4B9\t1027241\n1030\t1C4EA\t969840\n1031\t1C51D\t1487F60\n1032\t1C54E\t3C7CA1\n1033\t1C581\tC27801\n1034\t1C5B2\t1147941\n1035\t1C5E5\t12C7DE1\n1036\t1C616\t1D873C0\n1037\t1C649\t1A29701\n1038\t1C67A\t1526D61\n1039\t1C6AD\tAA8380\n1040\t1C6DE\t388BE0\n1041\t1C711\tA46A20\n1042\t1C742\tD49BE0\n1043\t1C775\t1A88361\n1044\t1C7A6\t1788081\n1045\t1C7D9\t1047FC1\n1046\t1C80A\t1B67F40\n1047\t1C83D\t487E41\n1048\t1C86E\t5A6D01\n1049\t1C8A1\t666D01\n1050\t1C8D2\t3679C1\n1051\t1C905\t10C68E1\n1052\t1C936\t1DC8821\n1053\t1C969\t1826CC1\n1054\t1C99A\t1D493A1\n1055\t1C9CD\t2A7720\n1056\t1C9FE\tF86F80\n1057\t1CA31\t45F40\n1058\t1CA62\tB29000\n1059\t1CA95\tE85D61\n1060\t1CAC6\t1387BA0\n1061\t1CAF9\t1847660\n1062\t1CB2A\t1366F20\n1063\t1CB5D\tC86DC0\n1064\t1CB8E\t3A6AC0\n1065\t1CBC1\t1867A20\n1066\t1CBF2\t1167800\n1067\t1CC25\t16C7401\n1068\t1CC56\t17C75E0\n1069\t1CC89\t1C465C0\n1070\t1CCBA\t1D67860\n1071\t1CCED\t6A7CC1\n1072\t1CD1E\t11C89C1\n1073\t1CD51\t828700\n1074\t1CD82\t3467A0\n1075\t1CDB5\t1AE5BE0\n1076\t1CDE6\t13CA241\n1077\t1CE19\t16275C1\n1078\t1CE4A\t15077C1\n1079\t1CE7D\tAE6D00\n1080\t1CEAE\tDC6200\n1081\t1CEE1\tA07AA1\n1082\t1CF12\t306FA0\n1083\t1CF45\t16A80E1\n1084\t1CF76\t19C8AE1\n1085\t1CFA9\t1A46261\n1086\t1CFDA\t17283E1\n1087\t1D00D\t8C63A1\n1088\t1D03E\t7C8E61\n1089\t1D071\t6284E0\n1090\t1D0A2\tD266A0\n1091\t1D0D5\t14E78E0\n1092\t1D106\t1DA6000\n1093\t1D139\t1227660\n1094\t1D16A\tF07721\n1095\t1D19D\tEE7281\n1096\t1D1CE\tBC69A1\n1097\t1D201\tE0B420\n1098\t1D232\tB06A80\n1099\t1D265\t18E7941\n1100\t1D296\t5C8D81\n1101\t1D2C9\t1427941\n1102\t1D2FA\t1928881\n1103\t1D32D\t286641\n1104\t1D35E\t9C9201\n1105\t1D391\t2085E1\n1106\t1D3C2\t7290A0\n1107\t1D3F5\tEC9CA1\n1108\t1D426\tFC6761\n1109\t1D459\t4077A1\n1110\t1D48A\t1906980\n1111\t1D4BD\t6E6A61\n1112\t1D4EE\t7081E0\n1113\t1D521\t427BE1\n1114\t1D552\t1D07A40\n1115\t1D585\t16E6CE1\n1116\t1D5B6\t748361\n1117\t1D5E9\t608640\n1118\t1D61A\t1327320\n1119\t1D64D\t2C9760\n1120\t1D67E\t7684E0\n1121\t1D6B1\t2069E0\n1122\t1D6E2\t1707640\n1123\t1D715\t12EB461\n1124\t1D746\t526F01\n1125\t1D779\t407261\n1126\t1D7AA\t1106660\n1127\t1D7DD\tCC70C1\n1128\t1D80E\t507661\n1129\t1D841\t2E7561\n1130\t1D872\t1B07A20\n1131\t1D8A5\t8E7200\n1132\t1D8D6\tB48601\n1133\t1D909\t10E79C1\n1134\t1D93A\t1309821\n1135\t1D96D\t4E5DE0\n1136\t1D99E\t9060A0\n1137\t1D9D1\tCE9800\n1138\t1DA02\tB66160\n1139\t1DA35\t207101\n1140\t1DA66\tD07060\n1141\t1DA99\t605600\n1142\t1DB5C\t46741\n1143\t1DB8F\t406741\n1144\t1DBC0\t206A61\n1145\t1DBF3\t607601\n1146\t1DC24\t46241\n1147\t1DC57\tE061C0\n1148\t1DCD6\t208C00\n1149\t1DD09\tA070C1\n1150\t1DD3A\t47000\n1151\t1DD6D\t406BA0\n1152\t1DD9E\t6072E1\n1153\t1DDD1\t207401\n1154\t1DF2A\t406080\n1155\t1DF5D\t2060E0\n1156\t1E17E\t2064E1\n1157\t1E39F\t406441\n1158\t1E500\t207720\n1159\t1E533\t1AE6140\n1160\t1E564\tE056C1\n1161\t1E597\t46A20\n1162\t1E5C8\t607181\n1163\t1E5FB\t4073E1\n1164\t1E62C\t205821\n1165\t1E677\t206061\n1166\t1EA42\t3C5B40\n1167\t1EF3D\t2E6AE1\n1168\t1EF6E\t1D06A41\n1169\t1EFA1\tE06580\n1170\t1EFD2\t306621\n1171\t1F005\t1AE70A1\n1172\t1F036\tF05E20\n1173\t1F069\t48C21\n1174\t1F09A\t507580\n1175\t1F0CD\tA06D61\n1176\t1F0FE\t208C41\n1177\t1F131\t607A80\n1178\t1F162\t46061\n1179\t1F195\t408B40\n1180\t1F1C6\t206EE1\n1181\t1F1F9\t6067C1\n1182\t1F22A\t206580\n1183\t1F261\tE06F61\n1184\t1F426\t1D07481\n1185\t1F459\t1AE6B40\n1186\t1F48A\t306D01\n1187\t1F4BD\t462A0\n1188\t1F4EE\tA06521\n1189\t1F521\t2089E1\n1190\t1F552\t406E21\n1191\t1F585\t606AE1\n1192\t1F5B6\t305BE0\n1193\t1F5E9\t45BA0\n1194\t1F61A\tE062E1\n1195\t1F64D\t208381\n1196\t1F67E\tA06521\n1197\t1F6B1\t407420\n1198\t1F6E2\t46A20\n1199\t1F715\t6053A0\n1200\t1F746\t208EE0\n1201\t1F779\t407681\n1202\t1F7AA\t207861\n1203\t1F8D3\t6076E0\n1204\t1F920\t207B01\n1205\t1F953\t406061\n1206\t1F9FC\t46B41\n1207\t1FA2F\t607800\n1208\t1FA60\t206FC1\n1209\t1FA93\t606480\n1210\t1FB26\t206760\n1211\t1FB59\tE06380\n1212\t1FC52\t47161\n1213\t1FC85\tA069A0\n1214\t1FCB6\t208820\n1215\t1FCE9\t406920\n1216\t1FD1A\t606D61\n1217\t1FD4D\t47041\n1218\t1FE0A\t406E00\n1219\t1FE3D\t207861\n1220\t1FE6E\t6063C0\n1221\t1FEA1\t45121\n1222\t1FFBE\t207041\n1223\t1FFF1\t4067E1\n1224\t20022\t46CA1\n1225\t20055\t207780\n1226\t20086\t6063A0\n1227\t200FF\t470A0\n1228\t20130\t406A40\n1229\t20163\t207E40\n1230\t20194\t606C21\n1231\t204BB\t46361\n1232\t204EC\t406721\n1233\t2051F\t207FC0\n1234\t20550\t1D07100\n1235\t2059B\t2E6E20\n1236\t205CC\t507580\n1237\t205FF\tE050C1\n1238\t20630\tD07900\n1239\t20663\t47BC1\n1240\t20694\t3076E0\n1241\t206C7\tA06E20\n1242\t206F8\t209BC0\n1243\t2072B\t606AE1\n1244\t2075C\t407820\n1245\t2078F\t206721\n1246\t207FA\t606220\n1247\t20889\t46821\n1248\t208BA\t207E80\n1249\t208ED\t386800\n1250\t209B2\t18E6DA0\n1251\t209E5\t1B06701\n1252\t20A16\tE08600\n1253\t20A49\t3C6FA0\n1254\t20A7A\t10E6F81\n1255\t20AAD\t326CC1\n1256\t20ADE\t49881\n1257\t20B11\t1D080A1\n1258\t20B42\t1AE61A1\n1259\t20B75\t906A00\n1260\t20BA6\tA08CC1\n1261\t20BD9\tF072E1\n1262\t20C0A\t2E7700\n1263\t20C3D\t707E20\n1264\t20C6E\t208E20\n1265\t20CA1\tD05CC1\n1266\t20CD2\t4097A0\n1267\t20D05\t308281\n1268\t20D36\t464C0\n1269\t20D69\t367A20\n1270\t20D9A\t6078C0\n1271\t20DCD\t506480\n1272\t20DFE\t207E01\n1273\t20E31\t1D06740\n1274\t20EAC\t18E6A20\n1275\t20EDF\t1DC6D20\n1276\t20F10\tE07140\n1277\t20F43\tD06481\n1278\t20F74\t2E72C0\n1279\t20FA7\tF062E0\n1280\t20FD8\t48840\n1281\t2100B\t3081C0\n1282\t2103C\t18E6141\n1283\t2106F\t1D06480\n1284\t210A0\tA07CC1\n1285\t210D3\tD06C40\n1286\t21104\t2E6A00\n1287\t21137\t1D08800\n1288\t21168\t2093C1\n1289\t2119B\t325020\n1290\t211CC\t18E7840\n1291\t211FF\t706DA0\n1292\t21230\tE06AE0\n1293\t21263\t3C7C80\n1294\t21294\t4E6180\n1295\t212C7\t1505F20\n1296\t212F8\t1C463C0\n1297\t2132B\t3467A0\n1298\t2135C\t1AE6EC1\n1299\t2138F\t1D87900\n1300\t213C0\t478C1\n1301\t213F3\t1D289C0\n1302\t21424\t2C6CA1\n1303\t21457\t3874A1\n1304\t21488\t1C65C61\n1305\t214BB\tB07FC0\n1306\t214EC\t14E6020\n1307\t2151F\t1DA7AA1\n1308\t21550\t407401\n1309\t21583\t1306A01\n1310\t215B4\tCE5A20\n1311\t215E7\tBC6F61\n1312\t21618\t1026280\n1313\t2164B\t3281C1\n1314\t2167C\t18E60C1\n1315\t216AF\t17C6220\n1316\t216E0\t205D00\n1317\t21713\t1926A81\n1318\t21744\t2E76C1\n1319\t21777\t7C6B60\n1320\t217A8\t1C26DE0\n1321\t217DB\t307781\n1322\t2180C\t16E64C1\n1323\t2183F\t1DC7B60\n1324\t21870\tE09160\n1325\t218A3\t1905B81\n1326\t218D4\tAE79E1\n1327\t21907\t5A70E0\n1328\t21938\t1A465A0\n1329\t2196B\t347CA0\n1330\t2199C\t1AE7421\n1331\t219CF\t3C6D40\n1332\t21A00\t47AC0\n1333\t21A33\t1D477E0\n1334\t21A64\t2E7C20\n1335\t21A97\tFC6CA0\n1336\t21AC8\tA07DE1\n1337\t21AFB\t905AA0\n1338\t21B2C\t18E6580\n1339\t21B5F\t1107EE1\n1340\t21B90\t20A760\n1341\t21BC3\t325E60\n1342\t21BF4\tEE71A0\n1343\t21C27\t1D66021\n1344\t21C58\tE07341\n1345\t21C8B\t367061\n1346\t21CBC\t6E8201\n1347\t21CEF\t1706761\n1348\t21D20\t207240\n1349\t21D53\t306BC1\n1350\t21D84\t2E7961\n1351\t21DB7\t3C7700\n1352\t21DE8\t608A61\n1353\t21E1B\t1D07561\n1354\t21E4C\t10E70C1\n1355\t21E7F\tD07A41\n1356\t21EB0\t47840\n1357\t21EE3\tF07561\n1358\t21F14\t8E7F40\n1359\t21F47\t706CA1\n1360\t21F78\tE079E1\n1361\t21FAB\t1B07400\n1362\t21FDC\t4E69A0\n1363\t2200F\t507040\n1364\t22040\t207AE1\n1365\t22073\t15076E1\n1366\t220A4\tA07241\n1367\t220D7\t46400\n1368\t22108\t4073C0\n1369\t2213B\t206FA1\n1370\t2216C\t605E40\n1371\t2219F\t45B41\n1372\t22230\t207541\n1373\t22263\t2058C0\n1374\t22294\t4058E1\n1375\t2236B\t208B01\n1376\t2239C\t2073A0\n1377\t225B1\t3C67A1\n1378\t225FE\t1AE5EC1\n1379\t22631\t326AA1\n1380\t22662\t1C260A0\n1381\t22695\t1D075C1\n1382\t226C6\t2E77A0\n1383\t226F9\t307B41\n1384\t2272A\tE07DC1\n1385\t2275D\t7074E0\n1386\t2278E\t18E6E21\n1387\t227C1\t506B80\n1388\t227F2\t48321\n1389\t22825\t4E7260\n1390\t22856\tA08301\n1391\t22889\t1D06B80\n1392\t228BA\t1AE69A0\n1393\t228ED\t3062A1\n1394\t2291E\t20A281\n1395\t22951\t506C41\n1396\t22982\t2E6BE0\n1397\t229B5\t1D06E40\n1398\t229E6\tE072C1\n1399\t22A19\t305E80\n1400\t22A4A\t18E62C0\n1401\t22A7D\t47A60\n1402\t22AAE\t1AE5AC0\n1403\t22AE1\t13C6B60\n1404\t22B12\t1C671A1\n1405\t22B45\t1306DE1\n1406\t22B76\tCE7960\n1407\t22BA9\t3888E0\n1408\t22BDA\t607421\n1409\t22C0D\t3480C0\n1410\t22C3E\t12E80C0\n1411\t22C71\t1D88C41\n1412\t22CA2\t1027080\n1413\t22CD5\t1B27641\n1414\t22D06\t2A5721\n1415\t22D39\t7A7740\n1416\t22D6A\t209361\n1417\t22D9D\tB08381\n1418\t22DCE\t18E8E01\n1419\t22E01\t1BC6FA0\n1420\t22E32\t1C45541\n1421\t22E65\t1908521\n1422\t22E96\tAE7BE0\n1423\t22EC9\t387C21\n1424\t22EFA\tE098C0\n1425\t22F2D\t328B80\n1426\t22F5E\t14E62A0\n1427\t22F91\t17C6E80\n1428\t22FC2\t1A47821\n1429\t22FF5\t1D686A1\n1430\t23026\t286240\n1431\t23059\t3A6E40\n1432\t2308A\t4A4A0\n1433\t230BD\t709001\n1434\t230EE\t1C877C0\n1435\t23121\t1DC9300\n1436\t23152\t1C27661\n1437\t23185\t967F40\n1438\t231B6\tEE7040\n1439\t231E9\t5A72C0\n1440\t2321A\tA0A420\n1441\t2324D\tD07461\n1442\t2327E\t16E7181\n1443\t232B1\t1DA7AC1\n1444\t232E2\t208FE1\n1445\t23315\t1D285C0\n1446\t23346\t2C6A80\n1447\t23379\t3C7501\n1448\t233AA\t407AA0\n1449\t233DD\t3095E1\n1450\t2340E\t1AE8601\n1451\t23441\tBC6AA1\n1452\t23472\t4A841\n1453\t234A5\t1705D61\n1454\t234D6\t6E77A1\n1455\t23509\t7C6661\n1456\t2353A\tE06680\n1457\t2356D\t907FE0\n1458\t2359E\t2E8D60\n1459\t235D1\tFC63E1\n1460\t23602\t206CE0\n1461\t23635\t1D09161\n1462\t23666\t10E9280\n1463\t23699\t5C58A1\n1464\t236CA\tA06740\n1465\t236FD\t367421\n1466\t2372E\t8E7520\n1467\t23761\tF08200\n1468\t23792\t47C00\n1469\t237C5\tD063E0\n1470\t237F6\t4E85E0\n1471\t23829\t1D48740\n1472\t2385A\t606240\n1473\t2388D\t307121\n1474\t238BE\t207801\n1475\t238F1\t1B06F00\n1476\t23922\tA06DA1\n1477\t23955\t707E01\n1478\t23986\t45DA0\n1479\t239B9\t1D077C0\n1480\t239EA\t4070E1\n1481\t23A1D\t305FC0\n1482\t23A4E\t2088C1\n1483\t23A81\t1109381\n1484\t23AB2\t607841\n1485\t23AE5\t5096A0\n1486\t23B16\t45DE1\n1487\t23B49\t1D47F21\n1488\t23B7A\t15079E1\n1489\t23BAD\t208B61\n1490\t23BDE\t1D47AA0\n1491\t23C11\t473A0\n1492\t23C42\t3C5AC0\n1493\t23D05\t2E6E01\n1494\t23D36\t326680\n1495\t23D69\tE062C0\n1496\t23D9A\t1D05840\n1497\t23DCD\t20BE01\n1498\t23DFE\t3075E0\n1499\t23E31\tA08141\n1500\t23E62\t1D482E0\n1501\t23E95\t48981\n1502\t23EC6\t706A20\n1503\t23EF9\t4082A1\n1504\t23F2A\t1D47500\n1505\t23F5D\t2080A0\n1506\t23F8E\t5071E1\n1507\t23FC1\t6076A1\n1508\t23FF2\t1D46661\n1509\t24093\t1D46F61\n1510\t240D0\t206980\n1511\t24121\t406B60\n1512\t241AE\t1D474E0\n1513\t241E1\t471E0\n1514\t24212\t1D05DE0\n1515\t24245\tE06EA0\n1516\t24276\t1D47021\n1517\t242A9\t207BC1\n1518\t242DA\t1D47761\n1519\t2430D\tA06761\n1520\t2433E\t46C01\n1521\t24371\t6062E0\n1522\t243A2\t206F80\n1523\t243D5\t4070A0\n1524\t24406\t1D45B81\n1525\t24439\t1D475C0\n1526\t244A0\t1B261E1\n1527\t245CB\t48BE0\n1528\t245FC\t1D48D80\n1529\t2462F\tE05B21\n1530\t24660\t206C40\n1531\t24693\t1D48B61\n1532\t246C4\t606D40\n1533\t246F7\t1D48000\n1534\t24728\t206A80\n1535\t2475B\t4054A0\n1536\t2478C\t1D05621\n1537\t247BF\t48420\n1538\t247F0\t1B270A0\n1539\t24823\tA066E1\n1540\t24854\t1D47041\n1541\t24887\t207AE1\n1542\t248B8\t606600\n1543\t248EB\t48041\n1544\t2491C\t1B27C21\n1545\t2494F\t407261\n1546\t24980\t1D47D80\n1547\t249B3\t208140\n1548\t249E4\t1D463E0\n1549\t24A17\t606240\n1550\t24A48\t3C6FC0\n1551\t24A7B\t18E5B60\n1552\t24AAC\t3060A0\n1553\t24ADF\t1C26BC1\n1554\t24B10\t1DC6740\n1555\t24B43\t4E6440\n1556\t24B74\t1306A61\n1557\t24BA7\t464E1\n1558\t24BD8\t386380\n1559\t24C0B\t16E6C81\n1560\t24C3C\t327021\n1561\t24C6F\t1C65DA0\n1562\t24CA0\t1D86E81\n1563\t24CD3\t2E5201\n1564\t24D04\t1D66C41\n1565\t24D37\tE079E1\n1566\t24D68\t3A6621\n1567\t24D9B\t1C86A60\n1568\t24DCC\t906440\n1569\t24DFF\t1C46701\n1570\t24E30\t1DC6B40\n1571\t24E63\tEE64A1\n1572\t24E94\t1906D41\n1573\t24EC7\t209721\n1574\t24EF8\t3C8520\n1575\t24F2B\t18E72A1\n1576\t24F5C\t707EA1\n1577\t24F8F\t1C27841\n1578\t24FC0\t1B27480\n1579\t24FF3\t8E6381\n1580\t25024\tD06800\n1581\t25057\tA07B60\n1582\t25088\tF076C1\n1583\t250BB\t1AE6C00\n1584\t250EC\t3081A0\n1585\t2511F\t48840\n1586\t25150\t1D07E60\n1587\t25183\t2E7841\n1588\t251B4\t366480\n1589\t251E7\t1C27A61\n1590\t25218\t1DC7520\n1591\t2524B\t12E6760\n1592\t2527C\t1707961\n1593\t252AF\tE09860\n1594\t252E0\t386A01\n1595\t25313\t10E7800\n1596\t25344\t346F40\n1597\t25377\t209721\n1598\t253A8\t5A75A1\n1599\t253DB\t18E7D20\n1600\t2540C\t1D27201\n1601\t2543F\t4085E1\n1602\t25470\t7C6AA1\n1603\t254A3\t2E7C80\n1604\t254D4\tB06B21\n1605\t25507\t4A901\n1606\t25538\t3C7BA0\n1607\t2556B\t16E7501\n1608\t2559C\t1107800\n1609\t255CF\tE066C1\n1610\t25600\t5C6A21\n1611\t25633\t6E63C1\n1612\t25664\t326F20\n1613\t25697\t206F20\n1614\t256C8\t3A78C0\n1615\t256FB\t1C86381\n1616\t2572C\t1D66021\n1617\t2575F\t1C474E1\n1618\t25790\t386160\n1619\t257C3\t2E6280\n1620\t257F4\t308961\n1621\t25827\tA08821\n1622\t25858\t3C5641\n1623\t2588B\t12E6CC1\n1624\t258BC\t1B057A1\n1625\t258EF\t1C26681\n1626\t25920\t327140\n1627\t25953\t4E7361\n1628\t25984\t1B27021\n1629\t259B7\t49561\n1630\t259E8\tD05D81\n1631\t25A1B\t18E6020\n1632\t25A4C\tF07EE1\n1633\t25A7F\tE06661\n1634\t25AB0\t708000\n1635\t25AE3\t2E6A41\n1636\t25B14\t1D08F01\n1637\t25B47\t206FE0\n1638\t25B78\t907361\n1639\t25BAB\t16E66C0\n1640\t25BDC\t386380\n1641\t25C0F\t1C26DA1\n1642\t25C40\t15075A0\n1643\t25C73\t10E6541\n1644\t25CA4\t3C6A60\n1645\t25CD7\t607920\n1646\t25D08\t326AE0\n1647\t25D3B\t1AE7821\n1648\t25D6C\t1D49020\n1649\t25D9F\t46BA0\n1650\t25DD0\t3070E0\n1651\t25E03\t2E65A0\n1652\t25E34\tF067A1\n1653\t25E67\tE07D40\n1654\t25E98\tD08B20\n1655\t25ECB\t12E5741\n1656\t25EFC\t1D690E1\n1657\t25F2F\t209860\n1658\t25F60\t507080\n1659\t25F93\t4E71A0\n1660\t25FC4\t19075C0\n1661\t25FF7\tA083C1\n1662\t26028\t907540\n1663\t2605B\t18E60A1\n1664\t2608C\t1B26741\n1665\t260BF\t207941\n1666\t260F0\t708C21\n1667\t26123\t2E85A1\n1668\t26154\t1D87E61\n1669\t26187\t1C66E60\n1670\t261B8\t1306741\n1671\t261EB\t14E6860\n1672\t2621C\t387220\n1673\t2624F\tE08DE0\n1674\t26280\t346B60\n1675\t262B3\tCE7720\n1676\t262E4\t1DC6B40\n1677\t26317\t1C46C00\n1678\t26348\t1D060E1\n1679\t2637B\t1C86DC1\n1680\t263AC\t5A6AA0\n1681\t263DF\t47921\n1682\t26410\tD07AE1\n1683\t26443\t8E6480\n1684\t26474\t3C7B00\n1685\t264A7\t1C28040\n1686\t264D8\t1706401\n1687\t2650B\t12E7900\n1688\t2653C\t3273C0\n1689\t2656F\t4062A0\n1690\t265A0\t1D260C1\n1691\t265D3\tEE6CC0\n1692\t26604\t307B00\n1693\t26637\t208120\n1694\t26668\t11069C0\n1695\t2669B\t18E7401\n1696\t266CC\t906F00\n1697\t266FF\tA084A0\n1698\t26730\t1D686A1\n1699\t26763\t4E73C1\n1700\t26794\t3668A1\n1701\t267C7\t474E0\n1702\t267F8\t1B06CE1\n1703\t2682B\t16E7020\n1704\t2685C\t5079A1\n1705\t2688F\t607F40\n1706\t268C0\t1B29040\n1707\t268F3\t10E75E0\n1708\t26924\tF08441\n1709\t26957\t1AE6560\n1710\t26988\t1D0A641\n1711\t269BB\t1506C61\n1712\t269EC\t1D47300\n1713\t26A1F\t19071E0\n1714\t26A50\t1D6A701\n1715\t26A83\t1D2A1C0\n1716\t26AB4\t1D07241\n1717\t26AE7\t1B2DFA0\n1718\t26B18\t1D68160\n1719\t26B4B\t1D27BA1\n1720\t26B7C\t1D075C1\n1721\t26BAF\t1B2D041\n1722\t26BE0\t1D6B020\n1723\t26C13\t207D20\n1724\t26C44\t3C6B01\n1725\t26C77\t406100\n1726\t26CA8\t308340\n1727\t26CDB\t47C21\n1728\t26D0C\t3C7F61\n1729\t26D3F\tE072C1\n1730\t26D70\t1D471C1\n1731\t26DA3\t209F61\n1732\t26DD4\t3C76A1\n1733\t26E07\tA06AC0\n1734\t26E38\tD05FA1\n1735\t26E6B\t46BA0\n1736\t26E9C\t3C7141\n1737\t26ECF\t607B21\n1738\t26F00\t1D06EC1\n1739\t26F33\t206B00\n1740\t26F64\t1B2D861\n1741\t26F97\t408FA0\n1742\t26FC8\t3CA2A1\n1743\t26FFB\t46D21\n1744\t2702C\t1D6AC00\n1745\t2705F\t6066A0\n1746\t27090\t3C6EA1\n1747\t270C3\t207B61\n1748\t270F4\t1D28A21\n1749\t27127\t4086A0\n1750\t27158\t3C64C1\n1751\t2718B\t1D091A1\n1752\t271BC\t3C7620\n1753\t271EF\t1D47E40\n1754\t27220\t3C9A21\n1755\t27253\t1D6DE00\n1756\t27284\t3C6DC1\n1757\t272B7\t208420\n1758\t272E8\t1D2D720\n1759\t2731B\t606740\n1760\t2734C\t3C83A1\n1761\t2737F\t406860\n1762\t273B0\t1D06261\n1763\t273E3\t2086E1\n1764\t27414\t3C6941\n1765\t27447\t406361\n1766\t27478\t1D465C1\n1767\t274AB\t207DA1\n1768\t274DC\t1D6CC41\n1769\t2750F\t1D2CDA0\n1770\t27540\t1D075E0\n1771\t27573\t2E7700\n1772\t275A4\t3C97E0\n1773\t275D7\t1C26A21\n1774\t27608\t326E00\n1775\t2763B\t18E6AA1\n1776\t2766C\t3C9660\n1777\t2769F\tE07D01\n1778\t276D0\t1B06120\n1779\t27703\t1AE6CE1\n1780\t27734\t3883E1\n1781\t27767\t1C471E1\n1782\t27798\t707000\n1783\t277CB\t6E5FA1\n1784\t277FC\t3C7A40\n1785\t2782F\t488C1\n1786\t27860\t1D46961\n1787\t27893\t14E6B60\n1788\t278C4\t3C8800\n1789\t278F7\t1C27441\n1790\t27928\t3473C0\n1791\t2795B\t2E8421\n1792\t2798C\t1DC61E0\n1793\t279BF\tA07AA1\n1794\t279F0\tF06BC1\n1795\t27A23\t18E7720\n1796\t27A54\t387521\n1797\t27A87\t20A5E0\n1798\t27AB8\tB056A1\n1799\t27AEB\tEE60A0\n1800\t27B1C\t1DC73C1\n1801\t27B4F\t1C66040\n1802\t27B80\t1D71740\n1803\t27BB3\t12E6F80\n1804\t27BE4\t5A6A60\n1805\t27C17\tE07B20\n1806\t27C48\t327C21\n1807\t27C7B\t2E8A20\n1808\t27CAC\t387600\n1809\t27CDF\t1C27620\n1810\t27D10\t1706E80\n1811\t27D43\t1AE6B40\n1812\t27D74\t3CC861\n1813\t27DA7\t495C1\n1814\t27DD8\t307320\n1815\t27E0B\tAE6481\n1816\t27E3C\t3CCCC0\n1817\t27E6F\t6082A0\n1818\t27EA0\t1D324A0\n1819\t27ED3\t16E6A21\n1820\t27F04\t3CC120\n1821\t27F37\t20AB00\n1822\t27F68\tD08000\n1823\t27F9B\t2E6840\n1824\t27FCC\t3CB4E1\n1825\t27FFF\tA08100\n1826\t28030\t11064C1\n1827\t28063\t18E6DE1\n1828\t28094\t3C81C0\n1829\t280C7\t408360\n1830\t280F8\t3673E0\n1831\t2812B\t10E69C0\n1832\t2815C\t3C71E1\n1833\t2818F\t45E81\n1834\t281C0\t1D08481\n1835\t281F3\t1AE65E1\n1836\t28224\t3C98C1\n1837\t28257\tA066A0\n1838\t28288\t9078A0\n1839\t282BB\t2E5E80\n1840\t282EC\t3C9960\n1841\t2831F\t209121\n1842\t28350\t1907E20\n1843\t28383\t4E6B01\n1844\t283B4\t3C9341\n1845\t283E7\t607640\n1846\t28418\t3067A1\n1847\t2844B\t2E60E1\n1848\t2847C\t3C7BA0\n1849\t284AF\t207A60\n1850\t284E0\t1D47960\n1851\t28513\t8E6AE1\n1852\t28544\t3C9780\n1853\t28577\tE065A1\n1854\t285A8\tD06020\n1855\t285DB\t207461\n1856\t2860C\t3C7DC0\n1857\t2863F\tA07961\n1858\t28670\tF07E00\n1859\t286A3\t206741\n1860\t286D4\t3C9000\n1861\t28707\tE07140\n1862\t28738\t707140\n1863\t2876B\t207820\n1864\t2879C\t3C91E0\n1865\t287CF\t4078A1\n1866\t28800\t1D05F00\n1867\t28833\t607CA1\n1868\t28864\t3C97A1\n1869\t28897\t207D61\n1870\t288C8\t306840\n1871\t288FB\t406A20\n1872\t2892C\t3CC440\n1873\t2895F\t606E80\n1874\t28990\t1506BC0\n1875\t289C3\t3CBFA1\n1876\t289F4\t2067C0\n1877\t28A27\t507620\n1878\t28A58\t606DA1\n1879\t28A8B\t3C8C20\n1880\t28ABC\t1D46C80\n1881\t28AEF\t3CC5A0\n1882\t28B20\t1B07860\n1883\t28B53\t3CA7C1\n1884\t28B84\t1D074C0\n1885\t28BB7\t3CE9A1\n1886\t28BE8\t3CDBE1\n1887\t28C1B\t3CE9E0\n1888\t28C60\t3CE9A1\n1889\t28CEF\t3CE320\n1890\t28D8A\t2E6740\n1891\t28DDB\t308700\n1892\t28E0C\t472C1\n1893\t28E3F\t3CEDE1\n1894\t28E70\tE05860\n1895\t28EA3\t1D07160\n1896\t28ED4\t208FC0\n1897\t28F07\t3D1240\n1898\t28F38\tA07481\n1899\t28F6B\t207880\n1900\t28F9C\t3CC9A0\n1901\t28FCF\t407EA1\n1902\t29000\t607260\n1903\t29033\t3CEBC0\n1904\t2910A\t3CFAA0\n1905\t29235\t3CF8E0\n1906\t2935E\t206CE0\n1907\t293EF\t2070A0\n1908\t294C6\t3D2CA0\n1909\t294F9\t207521\n1910\t2952A\t206FA1\n1911\t295A7\t3D12A1\n1912\t295D8\t2069E0\n1913\t2968F\t3D0741\n1914\t296C0\tA06220\n1915\t296F3\t207DA1\n1916\t29724\t406C80\n1917\t29757\t207BC1\n1918\t29788\tE06160\n1919\t297BB\t606A60\n1920\t297EC\t705E60\n1921\t29839\t1AE68C1\n1922\t2986A\t3D4780\n1923\t2989D\t1C263E1\n1924\t298CE\t1D6F701\n1925\t29901\t2E6D80\n1926\t29932\t307281\n1927\t29965\t47280\n1928\t29996\t1D07CA1\n1929\t299C9\tE06D81\n1930\t299FA\t506FC0\n1931\t29A2D\t209A80\n1932\t29A5E\tA07881\n1933\t29A91\t4079E1\n1934\t29AC2\t206AC1\n1935\t29AF5\t607D81\n1936\t29B26\t206601\n1937\t29BAF\t2059E0\n1938\t29D6C\t1D70320\n1939\t29D9F\t206340\n1940\t29E6C\t2065E0\n1941\t29F2B\t606220\n1942\t2A0E8\t1D6FB80\n1943\t2A11B\t206100\n1944\t2A14C\t405901\n1945\t2A2A5\t1D70320\n1946\t2A2D6\t208041\n1947\t2A309\t606C41\n1948\t2A33A\t207041\n1949\t2A465\t1D6EC01\n1950\t2A496\t4058A0\n1951\t2A621\t1D70860\n1952\t2A652\t206D00\n1953\t2A685\t606B40\n1954\t2A6B6\t1D71500\n1955\t2A733\t47720\n1956\t2A764\tE05EE1\n1957\t2A797\t208360\n1958\t2A7C8\t905861\n1959\t2A7FB\t1AE6541\n1960\t2A82C\t1D06DE0\n1961\t2A85F\t1C47661\n1962\t2A890\t307640\n1963\t2A8C3\t2E6A41\n1964\t2A8F4\t1D6F140\n1965\t2A927\tA07141\n1966\t2A958\t705841\n1967\t2A98B\t46A61\n1968\t2A9BC\t506B20\n1969\t2A9EF\tE07541\n1970\t2AA20\t206A61\n1971\t2AA53\t406E00\n1972\t2AA84\t607441\n1973\t2AAB7\t207921\n1974\t2AB40\t1D6DA61\n1975\t2AB73\t207360\n1976\t2ABA4\t606060\n1977\t2ABD7\t1D6DD00\n1978\t2AC08\t2078E0\n1979\t2AC3B\t3071C0\n1980\t2ACFA\t2E7661\n1981\t2AD2D\t1D70B81\n1982\t2AD5E\tE065C1\n1983\t2AD91\t5066A0\n1984\t2ADC2\t47AE1\n1985\t2ADF5\t1D6E781\n1986\t2AE26\tA07460\n1987\t2AE59\t20A160\n1988\t2AE8A\t4075E1\n1989\t2AEBD\t306AA0\n1990\t2AEEE\t2E6CC0\n1991\t2AF21\t1D078C0\n1992\t2AF52\t46FA1\n1993\t2AF85\t706D00\n1994\t2AFB6\tE05860\n1995\t2AFE9\t1D6BE60\n1996\t2B01A\t208AC0\n1997\t2B04D\t506FC0\n1998\t2B07E\t18E5C20\n1999\t2B0B1\t1DC6C00\n2000\t2B0E2\tA06161\n2001\t2B115\tF07001\n2002\t2B146\t4E6B20\n2003\t2B179\t326961\n2004\t2B1AA\t46FC1\n2005\t2B1DD\t1D072A0\n2006\t2B20E\t1AE55E1\n2007\t2B241\tD07C00\n2008\t2B272\tE07900\n2009\t2B2A5\tF06B80\n2010\t2B2D6\t2E6420\n2011\t2B309\t326DA0\n2012\t2B33A\t2093A1\n2013\t2B36D\t1D6DD81\n2014\t2B39E\t10E63E1\n2015\t2B3D1\t3085E0\n2016\t2B402\t6078C0\n2017\t2B435\t1DC74E1\n2018\t2B466\t18E7701\n2019\t2B499\t17068C1\n2020\t2B4CA\t473A0\n2021\t2B4FD\t9066C0\n2022\t2B52E\t2E7301\n2023\t2B561\t1D07661\n2024\t2B592\tE08C00\n2025\t2B5C5\t326A01\n2026\t2B5F6\t1C86341\n2027\t2B629\tF06CA0\n2028\t2B65A\t1C47C01\n2029\t2B68D\t707820\n2030\t2B6BE\t4E6840\n2031\t2B6F1\t1B33C00\n2032\t2B722\t20A1C0\n2033\t2B755\tD063A1\n2034\t2B786\t18E6D41\n2035\t2B7B9\t1D69101\n2036\t2B7EA\tA06A21\n2037\t2B81D\t306F81\n2038\t2B84E\t2E6C81\n2039\t2B881\t1D38A01\n2040\t2B8B2\t47E61\n2041\t2B8E5\t906E40\n2042\t2B916\t1AE6261\n2043\t2B949\t3A67C1\n2044\t2B97A\t1C26681\n2045\t2B9AD\t1B07160\n2046\t2B9DE\t2E7C20\n2047\t2BA11\t366A21\n2048\t2BA42\tE069C1\n2049\t2BA75\t1D06F41\n2050\t2BAA6\t18E6D00\n2051\t2BAD9\t306761\n2052\t2BB0A\t2090A1\n2053\t2BB3D\t1B318C0\n2054\t2BB6E\t2E6461\n2055\t2BBA1\t706CA1\n2056\t2BBD2\t407A21\n2057\t2BC05\t1D6CFE1\n2058\t2BC36\t480C0\n2059\t2BC69\t507580\n2060\t2BC9A\t1AE5420\n2061\t2BCCD\t3A7460\n2062\t2BCFE\tE073E1\n2063\t2BD31\t1D37200\n2064\t2BD62\t2E6120\n2065\t2BD95\t307121\n2066\t2BDC6\t206C61\n2067\t2BDF9\t1D07741\n2068\t2BE2A\t18E6A40\n2069\t2BE5D\t7051E1\n2070\t2BE8E\tA06C60\n2071\t2BEC1\t1B31020\n2072\t2BEF2\t2E66C0\n2073\t2BF25\t306F00\n2074\t2BF56\t47C60\n2075\t2BF89\t1D69081\n2076\t2BFBA\tE064C0\n2077\t2BFED\t366C81\n2078\t2C01E\t204FE1\n2079\t2C051\t1B2F281\n2080\t2C082\t606A60\n2081\t2C0B5\t506FA0\n2082\t2C0E6\t207921\n2083\t2C119\t1D68301\n2084\t2C14A\t407FA0\n2085\t2C17D\t1B2E440\n2086\t2C1AE\t207F60\n2087\t2C1E1\t305641\n2088\t2C212\tE071A1\n2089\t2C245\t1D06201\n2090\t2C276\t46DE1\n2091\t2C2A9\t1D33820\n2092\t2C2DA\tA07181\n2093\t2C30D\t1D6A140\n2094\t2C33E\t208560\n2095\t2C371\t1B30B40\n2096\t2C3A2\t604BC0\n2097\t2C3D5\t1D06600\n2098\t2C406\t406FC1\n2099\t2C439\t1D32860\n2100\t2C46A\t2068E1\n2101\t2C49D\t1D683A1\n2102\t2C4CE\tE065C1\n2103\t2C501\t506A60\n2104\t2C532\t45D21\n2105\t2C565\t1B2E180\n2106\t2C596\tA06BC1\n2107\t2C5C9\t1D07001\n2108\t2C5FA\t208240\n2109\t2C62D\t1D692A1\n2110\t2C65E\t606E20\n2111\t2C691\t1B2D621\n2112\t2C6C2\t207000\n2113\t2C6F5\t1D67D41\n2114\t2C726\t4069E0\n2115\t2C759\t1D31501\n2116\t2C78A\t206301\n2117\t2C7BD\t1D68D60\n2118\t2C7EE\t606560\n2119\t2C821\t1B2E3A0\n2120\t2C852\t206E81\n2121\t2C885\tD06B81\n2122\t2C8B6\t6067A1\n2123\t2C8E9\t1D68BC0\n2124\t2C91A\t1B2C1E1\n2125\t2C94D\t1D68CC1\n2126\t2C97E\t207240\n2127\t2C9B1\t1D693A0\n2128\t2C9E2\t1D697E0\n2129\t2CA23\t1B2CB00\n2130\t2CA54\t1D68661\n2131\t2CA87\t1D30C21\n2132\t2CABE\t2E7320\n2133\t2CAF1\tD07981\n2134\t2CB22\tE06980\n2135\t2CB55\t1D6A4C1\n2136\t2CB86\t47560\n2137\t2CBB9\t1B2DA41\n2138\t2CBEA\tA07020\n2139\t2CC1D\t1D695E1\n2140\t2CC4E\t208420\n2141\t2CC81\t1D2D3E1\n2142\t2CCB2\t4073E1\n2143\t2CCE5\t1D6A081\n2144\t2CD16\t2082E0\n2145\t2CD49\t1B29940\n2146\t2CD7A\t606C00\n2147\t2CDAD\t1D68260\n2148\t2CDDE\t1D2D5E1\n2149\t2CE11\t1D68C40\n2150\t2CE42\t1B2A2A0\n2151\t2CE75\t1D674A0\n2152\t2CEA6\t1D2DB61\n2153\t2CED9\t1D692E0\n2154\t2CF0A\t1B2A800\n2155\t2CF3D\t1D68980\n2156\t2CF6E\t1D2B560\n2157\t2CFA1\t1D66F41\n2158\t2CFD2\t2070E1\n2159\t2D005\t1B2CDE1\n2160\t2D036\t1D67FE0\n2161\t2D069\t207780\n2162\t2D09A\t1D2A061\n2163\t2D0CD\t1D69CC0\n2164\t2D0FE\t406D81\n2165\t2D131\t1B2BAC0\n2166\t2D162\t46661\n2167\t2D195\t1D68800\n2168\t2D1C6\t605FC0\n2169\t2D1F9\t1D2BAC0\n2170\t2D22A\t207B01\n2171\t2D25D\t1D66E61\n2172\t2D28E\t1B2AF80\n2173\t2D2C1\t207DC1\n2174\t2D2F2\t1D68DE1\n2175\t2D325\t1D2CFC1\n2176\t2D356\t2072E0\n2177\t2D389\t1D677E1\n2178\t2D3BA\t1B2AFA1\n2179\t2D3ED\t207820\n2180\t2D41E\t1D68B00\n2181\t2D451\t1D2C580\n2182\t2D482\tE064A0\n2183\t2D4B5\t1D68421\n2184\t2D4E6\t46DA0\n2185\t2D519\t1B2AD60\n2186\t2D54A\tA076A1\n2187\t2D57D\t1D67A20\n2188\t2D5AE\t209080\n2189\t2D5E1\t1D2CDA0\n2190\t2D612\t407581\n2191\t2D645\t1D68400\n2192\t2D676\t462A0\n2193\t2D6A9\t1B27820\n2194\t2D6DA\t607361\n2195\t2D70D\t1D67421\n2196\t2D73E\t1D2CF61\n2197\t2D771\t2076A0\n2198\t2D7A2\t1D67C61\n2199\t2D7D5\t1B28280\n2200\t2D806\t2E5E01\n2201\t2D839\t1D68680\n2202\t2D86A\tA06C60\n2203\t2D89D\t1D2CEE1\n2204\t2D8CE\t476C0\n2205\t2D901\t1D67481\n2206\t2D932\t407541\n2207\t2D965\t1B29A61\n2208\t2D996\t209781\n2209\t2D9C9\t706721\n2210\t2D9FA\t2E6440\n2211\t2DA2D\t1D07221\n2212\t2DA5E\tE07321\n2213\t2DA91\tD07041\n2214\t2DAC2\t46FA1\n2215\t2DAF5\t1B067E0\n2216\t2DB26\t1AE6EE0\n2217\t2DB59\t3267E1\n2218\t2DB8A\t1C26F00\n2219\t2DBBD\t1D2A501\n2220\t2DBEE\t2E6BA1\n2221\t2DC21\t307800\n2222\t2DC52\tA06820\n2223\t2DC85\t1D67061\n2224\t2DCB6\t18E66A1\n2225\t2DCE9\tD06BE1\n2226\t2DD1A\t20A0A1\n2227\t2DD4D\t1B060C0\n2228\t2DD7E\t2E6CA0\n2229\t2DDB1\t5068E0\n2230\t2DDE2\tE07280\n2231\t2DE15\t1B26DE1\n2232\t2DE46\t1AE6C81\n2233\t2DE79\t3077E1\n2234\t2DEAA\t47521\n2235\t2DEDD\t1D06081\n2236\t2DF0E\t607F61\n2237\t2DF41\t706860\n2238\t2DF72\t20A1A0\n2239\t2DFA5\t1D27761\n2240\t2DFD6\tA075C1\n2241\t2E009\t1D66B20\n2242\t2E03A\t205A01\n2243\t2E06D\t1B28F21\n2244\t2E09E\t4079C0\n2245\t2E0D1\t1D67260\n2246\t2E102\t207FC0\n2247\t2E135\t1D27180\n2248\t2E166\tA06660\n2249\t2E199\t1B29221\n2250\t2E1CA\t6060A0\n2251\t2E1FD\t1D67020\n2252\t2E22E\t467C0\n2253\t2E261\t1D29620\n2254\t2E292\t406680\n2255\t2E2C5\t1B28041\n2256\t2E2F6\t206FE0\n2257\t2E329\t1D26A80\n2258\t2E35A\t606720\n2259\t2E38D\t1B29421\n2260\t2E3BE\t2E6021\n2261\t2E3F1\t307800\n2262\t2E422\t44E40\n2263\t2E455\t1D07460\n2264\t2E486\tA065A0\n2265\t2E4B9\t507F20\n2266\t2E4EA\t207BE0\n2267\t2E51D\t1D278E0\n2268\t2E54E\t4076C0\n2269\t2E581\t7065A1\n2270\t2E5B2\t207E01\n2271\t2E5E5\t1D680A1\n2272\t2E616\t6079A1\n2273\t2E649\t1B26E81\n2274\t2E67A\t407360\n2275\t2E6AD\t1D27641\n2276\t2E6DE\t1B264E1\n2277\t2E757\t1D28D20\n2278\t2E788\t1B260A1\n2279\t2E7BB\t2E6541\n2280\t2E7EC\t306941\n2281\t2E81F\t47541\n2282\t2E850\t1D28240\n2283\t2E883\tE07A81\n2284\t2E8B4\t1B27900\n2285\t2E8E7\t209100\n2286\t2E918\t1D26961\n2287\t2E94B\tA07CC1\n2288\t2E97C\t1B26E41\n2289\t2E9AF\t477A1\n2290\t2E9E0\t1D272E0\n2291\t2EA13\t607080\n2292\t2EA44\t1D275C0\n2293\t2EA77\t207F21\n2294\t2EAA8\t407FC0\n2295\t2EADB\t1D27180\n2296\t2EB26\t2082C1\n2297\t2EB59\t1B27461\n2298\t2EB8A\tA05F21\n2299\t2EBBD\t1D284C1\n2300\t2EBEE\t46BC0\n2301\t2EC21\t6068E0\n2302\t2EC52\t407F60\n2303\t2EC85\t505840\n2304\t2ECB6\t2086C0\n2305\t2ECE9\t1B261E1\n2306\t2ED1A\tE06760\n2307\t2ED4D\t307421\n2308\t2ED7E\t46D81\n2309\t2EDB1\t1D29620\n2310\t2EDE2\tA06480\n2311\t2EE15\t2076A0\n2312\t2EE46\t1D273E1\n2313\t2EE79\t606461\n2314\t2EEAA\t207FC0\n2315\t2EEDD\t1D268C0\n2316\t2EF0E\t406CE0\n2317\t2EF41\t1D264E1\n2318\t2EF8E\t207AC0\n2319\t2EFC1\t6065E1\n2320\t2EFF2\t1D85F01\n2321\t2F025\t12E7820\n2322\t2F056\t906500\n2323\t2F089\t1C273E0\n2324\t2F0BA\t1DC7620\n2325\t2F0ED\t10E6981\n2326\t2F11E\tF07800\n2327\t2F151\t47AC0\n2328\t2F182\t326EC0\n2329\t2F1B5\t18E7420\n2330\t2F1E6\t1D07040\n2331\t2F219\tE08E20\n2332\t2F24A\t1DC6DC1\n2333\t2F27D\t2E75C1\n2334\t2F2AE\t707761\n2335\t2F2E1\t209CC1\n2336\t2F312\t1706A21\n2337\t2F345\t1AE6E80\n2338\t2F376\t326C61\n2339\t2F3A9\tA07D21\n2340\t2F3DA\t1B25241\n2341\t2F40D\t2E70C1\n2342\t2F43E\tD07C41\n2343\t2F471\t47381\n2344\t2F4A2\t1B06F21\n2345\t2F4D5\t1AE5C00\n2346\t2F506\t3074E1\n2347\t2F539\tE07E20\n2348\t2F56A\t1D06960\n2349\t2F59D\t209D00\n2350\t2F5CE\t5061E0\n2351\t2F601\t408880\n2352\t2F632\t1D28681\n2353\t2F665\t2E56E1\n2354\t2F696\t3077A0\n2355\t2F6C9\t46221\n2356\t2F6FA\t387AC0\n2357\t2F72D\t14E6FE0\n2358\t2F75E\t1306EC0\n2359\t2F791\t1C66BA0\n2360\t2F7C2\t1D86AC1\n2361\t2F7F5\tAE59A1\n2362\t2F826\t329040\n2363\t2F859\tE05CC1\n2364\t2F88A\tFC7CE0\n2365\t2F8BD\t18E7761\n2366\t2F8EE\t1D08400\n2367\t2F921\t1C46D20\n2368\t2F952\t1DA62E0\n2369\t2F985\t2E86C1\n2370\t2F9B6\t908501\n2371\t2F9E9\t207A60\n2372\t2FA1A\t3D4581\n2373\t2FA4D\t16E5EC1\n2374\t2FA7E\t1507840\n2375\t2FAB1\tA069E1\n2376\t2FAE2\t1DC7301\n2377\t2FB15\tEE7601\n2378\t2FB46\t7063E0\n2379\t2FB79\t206841\n2380\t2FBAA\t5A72C0\n2381\t2FBDD\t1AE6820\n2382\t2FC0E\t1B26B81\n2383\t2FC41\tE07180\n2384\t2FC72\t3D2761\n2385\t2FCA5\t2E7841\n2386\t2FCD6\t325AE0\n2387\t2FD09\t1C66920\n2388\t2FD3A\t1DC5F60\n2389\t2FD6D\t18E6881\n2390\t2FD9E\t11078C0\n2391\t2FDD1\t470A0\n2392\t2FE02\t386361\n2393\t2FE35\t4E7F40\n2394\t2FE66\tD05501\n2395\t2FE99\t1C279C1\n2396\t2FECA\t3D3721\n2397\t2FEFD\t1AE7B60\n2398\t2FF2E\t1D07421\n2399\t2FF61\t6082E1\n2400\t2FF92\t3D1960\n2401\t2FFC5\t2E8160\n2402\t2FFF6\t3083E0\n2403\t30029\t209640\n2404\t3005A\t3CDFE0\n2405\t3008D\t10E7301\n2406\t300BE\t19069A1\n2407\t300F1\tE072C1\n2408\t30122\t3CFCE1\n2409\t30155\t8E71A0\n2410\t30186\t366CC0\n2411\t301B9\t47060\n2412\t301EA\t3D07C0\n2413\t3021D\tA07F80\n2414\t3024E\t1D466A1\n2415\t30281\t407240\n2416\t302B2\t3CD141\n2417\t302E5\t2060E0\n2418\t30316\t707F60\n2419\t30349\t3CB860\n2420\t3037A\t405B60\n2421\t303AD\tF07301\n2422\t303DE\t206441\n2423\t30411\t3CB361\n2424\t30442\t509220\n2425\t30475\t3CA0E1\n2426\t304A6\t1D28B80\n2427\t304D9\t3CC240\n2428\t3050A\t1707380\n2429\t3053D\t3CD6C1\n2430\t3056E\t1B07961\n2431\t305A1\t3CCD80\n2432\t305D2\t3C9180\n2433\t30607\t3C9161\n2434\t30638\t3CBCC1\n2435\t3066B\t3C63E1\n2436\t3069C\t18E65E0\n2437\t306CF\t326881\n2438\t30700\t1C263E1\n2439\t30733\t387B40\n2440\t30764\t2E6FA0\n2441\t30797\t1D07680\n2442\t307C8\tE079A0\n2443\t307FB\t3CD6E0\n2444\t3082C\t1AE7340\n2445\t3085F\t307C40\n2446\t30890\t483A0\n2447\t308C3\t3C8EE1\n2448\t308F4\tA07361\n2449\t30927\t707840\n2450\t30958\t20AEA0\n2451\t3098B\t3CA581\n2452\t309BC\t6095E1\n2453\t309EF\t507221\n2454\t30A20\t46AC1\n2455\t30A53\t3CAC81\n2456\t30A84\tA060E1\n2457\t30AB7\t3C7D81\n2458\t30AE8\t2080A0\n2459\t30B1B\t3C7B41\n2460\t30B4C\t2E7320\n2461\t30B7F\t1D06880\n2462\t30BB0\t1C27100\n2463\t30BE3\t3CCCC0\n2464\t30C14\t18E54A0\n2465\t30C47\t307F01\n2466\t30C78\tE07300\n2467\t30CAB\t3C8800\n2468\t30CDC\t1AE6EC1\n2469\t30D0F\t505DC1\n2470\t30D40\t47A41\n2471\t30D73\t3C7F80\n2472\t30DA4\t407DC1\n2473\t30DD7\t3CAB01\n2474\t30E08\t2094A0\n2475\t30E3B\t1B070A1\n2476\t30E6C\t4E62A1\n2477\t30E9F\t3C7340\n2478\t30ED0\t1C26D01\n2479\t30F03\t3079E0\n2480\t30F34\t2E6761\n2481\t30F67\t3C81A0\n2482\t30F98\tE062E1\n2483\t30FCB\t1D077A0\n2484\t30FFC\t12E6540\n2485\t3102F\t1DC69C0\n2486\t31060\t1C66CA1\n2487\t31093\t3265A1\n2488\t310C4\tCE6181\n2489\t310F7\t387280\n2490\t31128\t46F61\n2491\t3115B\tF07D00\n2492\t3118C\t18E7140\n2493\t311BF\t3A7781\n2494\t311F0\t1C27CC1\n2495\t31223\t906101\n2496\t31254\t2E7D81\n2497\t31287\t3C7781\n2498\t312B8\tA05DC1\n2499\t312EB\t1D08001\n2500\t3131C\t1AE6BE0\n2501\t3134F\t3C7821\n2502\t31380\t209EC0\n2503\t313B3\t325281\n2504\t313E4\t4E6B61\n2505\t31417\t1D86F61\n2506\t31448\t1A46120\n2507\t3147B\t1507900\n2508\t314AC\t14E5961\n2509\t314DF\t3876A0\n2510\t31510\tE08D20\n2511\t31543\t706601\n2512\t31574\t2E91C1\n2513\t315A7\t1DA6240\n2514\t315D8\t1C477A0\n2515\t3160B\t1D07EE1\n2516\t3163C\t18E6AE0\n2517\t3166F\tFC65A0\n2518\t316A0\t47541\n2519\t316D3\t346640\n2520\t31704\tEE7340\n2521\t31737\t1DC6A21\n2522\t31768\t1C26A21\n2523\t3179B\t1307360\n2524\t317CC\t12E5D21\n2525\t317FF\t5C7C20\n2526\t31830\t607241\n2527\t31863\tD065C1\n2528\t31894\t2E6C81\n2529\t318C7\t5A6021\n2530\t318F8\t20B8A1\n2531\t3192B\t19073A0\n2532\t3195C\t1C85921\n2533\t3198F\t3C9840\n2534\t319C0\tE06DA0\n2535\t319F3\t3274E0\n2536\t31A24\t8E6B80\n2537\t31A57\t3C6440\n2538\t31A88\t1C270C1\n2539\t31ABB\t1D46E81\n2540\t31AEC\t16E6C21\n2541\t31B1F\t1D87681\n2542\t31B50\t47000\n2543\t31B83\t3072E1\n2544\t31BB4\t2E8601\n2545\t31BE7\t3C6F81\n2546\t31C18\tA07901\n2547\t31C4B\tF09420\n2548\t31C7C\t18E65A1\n2549\t31CAF\t3C67E0\n2550\t31CE0\t1C266E1\n2551\t31D13\t3274A1\n2552\t31D44\tCE7681\n2553\t31D77\t3C8A20\n2554\t31DA8\t208140\n2555\t31DDB\t1D07400\n2556\t31E0C\t1AE8B00\n2557\t31E3F\t3876C0\n2558\t31E70\t1C46461\n2559\t31EA3\tB06F61\n2560\t31ED4\t2E7620\n2561\t31F07\t1DA61A1\n2562\t31F38\tE08820\n2563\t31F6B\t1707940\n2564\t31F9C\t12A55A0\n2565\t31FCF\tDC7A81\n2566\t32000\t1A659C1\n2567\t32033\tF28321\n2568\t32064\t6E66E0\n2569\t32097\t1987200\n2570\t320C8\t627220\n2571\t320FB\t1B47921\n2572\t3212C\tEC6C40\n2573\t3215F\t1187F21\n2574\t32190\t1626660\n2575\t321C3\t367940\n2576\t321F4\t4C5CC1\n2577\t32227\t15C6B60\n2578\t32258\t407880\n2579\t3228B\t1328561\n2580\t322BC\t14C5DE0\n2581\t322EF\tBA7A81\n2582\t32320\t1C660A1\n2583\t32353\t547A41\n2584\t32384\t10E8520\n2585\t323B7\t9851E1\n2586\t323E8\tA28FE1\n2587\t3241B\t1525F00\n2588\t3244C\t10A7E61\n2589\t3247F\tD88940\n2590\t324B0\t12456A1\n2591\t324E3\t1127941\n2592\t32514\tAC8FE0\n2593\t32547\t17A4CE0\n2594\t32578\tC67EE1\n2595\t325AB\t1B65CE1\n2596\t325DC\t18C87C0\n2597\t3260F\t7A79A0\n2598\t32640\tE666E0\n2599\t32673\t948621\n2600\t326A4\tA88041\n2601\t326D7\t1586C00\n2602\t32708\t847E21\n2603\t3273B\t1D256E0\n2604\t3276C\t1288280\n2605\t3279F\t587321\n2606\t327D0\t1847801\n2607\t32803\tF4A481\n2608\t32834\t8A7801\n2609\t32867\t15A79C0\n2610\t32898\tA67561\n2611\t328CB\t965B40\n2612\t328FC\t14A9140\n2613\t3292F\tDA6221\n2614\t32960\tE46DA1\n2615\t32993\t347081\n2616\t329C4\tCA7080\n2617\t329F7\t13A8140\n2618\t32A28\t267BA1\n2619\t32A5B\t1D66B20\n2620\t32A8C\t1A88040\n2621\t32ABF\t386C80\n2622\t32AF0\t1446C80\n2623\t32B23\t1148C60\n2624\t32B54\t285AA0\n2625\t32B87\t1BA6A81\n2626\t32BB8\t1668560\n2627\t32BEB\t1567F21\n2628\t32C1C\t12A8A40\n2629\t32C4F\t9A6CC0\n2630\t32C80\t10663E0\n2631\t32CB3\tB29041\n2632\t32CE4\t4876A1\n2633\t32D17\t1B87BC1\n2634\t32D48\t246C81\n2635\t32D7B\t1B265C1\n2636\t32DAC\tE869E1\n2637\t32DDF\tB87CA1\n2638\t32E10\t1047781\n2639\t32E43\t5681C0\n2640\t32E74\t4A6A40\n2641\t32EA7\t19A7981\n2642\t32ED8\t667460\n2643\t32F0B\t1368060\n2644\t32F3C\t18A7920\n2645\t32F6F\t3A7020\n2646\t32FA0\t1C66BA0\n2647\t32FD3\tD471C0\n2648\t33004\t16857E0\n2649\t33037\t788940\n2650\t33068\t646C20\n2651\t3309B\t19468E0\n2652\t330CC\t1088340\n2653\t330FF\t11A7540\n2654\t33130\t1C27A20\n2655\t33163\t1168A20\n2656\t33194\t6C72A0\n2657\t331C7\t1DC7841\n2658\t331F8\tC278E0\n2659\t3322B\t1967720\n2660\t3325C\t1AA6980\n2661\t3328F\tFC6660\n2662\t332C0\t1467E41\n2663\t332F3\t927BE0\n2664\t33324\t8875E0\n2665\t33357\t1788DA1\n2666\t33388\t472C1\n2667\t333BB\t1D47D20\n2668\t333EC\tEA7401\n2669\t3341F\tF867C0\n2670\t33450\t1027B60\n2671\t33483\tF677E1\n2672\t334B4\t2A6F40\n2673\t334E7\t1D87900\n2674\t33518\t866121\n2675\t3354B\tB68401\n2676\t3357C\t12C8121\n2677\t335AF\t3C7881\n2678\t335E0\t1267C80\n2679\t33613\t326661\n2680\t33644\tC87440\n2681\t33677\t1388B00\n2682\t336A8\tA475C0\n2683\t336DB\t1548D00\n2684\t3370C\t1C860C0\n2685\t3373F\t11879A0\n2686\t33770\t1A27E60\n2687\t337A3\tD673C0\n2688\t337D4\tAA8540\n2689\t33807\t1BC7B81\n2690\t33838\t18664E0\n2691\t3386B\t1769000\n2692\t3389C\t14C8040\n2693\t338CF\tFA87A0\n2694\t33900\t1A68500\n2695\t33933\t745B40\n2696\t33964\t6879C0\n2697\t33997\t1988620\n2698\t339C8\t446D20\n2699\t339FB\t1728A41\n2700\t33A2C\t1886C61\n2701\t33A5F\t587B01\n2702\t33A90\t1648100\n2703\t33AC3\t507160\n2704\t33AF4\t4C8B20\n2705\t33B27\t15C6320\n2706\t33B58\t4676A0\n2707\t33B8B\t1348CC1\n2708\t33BBC\t16C70C0\n2709\t33BEF\t7C7EE0\n2710\t33C20\tE26921\n2711\t33C53\t726461\n2712\t33C84\t1487F21\n2713\t33CB7\t986E21\n2714\t33CE8\tA27401\n2715\t33D1B\t1527B60\n2716\t33D4C\t18E5B41\n2717\t33D7F\t11C8121\n2718\t33DB0\t1C26140\n2719\t33DE3\t7670E1\n2720\t33E14\t6A71C0\n2721\t33E47\t17A64A1\n2722\t33E78\tE0A400\n2723\t33EAB\t1B07821\n2724\t33EDC\t10C6421\n2725\t33F0F\tBC7D40\n2726\t33F40\t1C665C1\n2727\t33F73\tD26761\n2728\t33FA4\tAE6E60\n2729\t33FD7\t13C65C1\n2730\t34008\t474E0\n2731\t3403B\t1D26FC1\n2732\t3406C\t14E6980\n2733\t3409F\t388440\n2734\t340D0\t1426241\n2735\t34103\t306761\n2736\t34134\t2C7500\n2737\t34167\t1D87060\n2738\t34198\tA07281\n2739\t341CB\t1107661\n2740\t341FC\t1AA6260\n2741\t3422F\t3C8881\n2742\t34260\tE259A0\n2743\t34293\t348EA1\n2744\t342C4\tCC6EA1\n2745\t342F7\t7863A0\n2746\t34328\t266821\n2747\t3435B\t1D665A0\n2748\t3438C\t1AE6840\n2749\t343BF\t11C81A0\n2750\t343F0\t18258E1\n2751\t34423\t907D00\n2752\t34454\t286720\n2753\t34487\t19C6980\n2754\t344B8\tE0B461\n2755\t344EB\t15069A1\n2756\t3451C\t16A91C0\n2757\t3454F\t9C7881\n2758\t34580\t1225BC0\n2759\t345B3\tF297E1\n2760\t345E4\t4E6B61\n2761\t34617\t17C78A0\n2762\t34648\t429480\n2763\t3467B\t1B47BC1\n2764\t346AC\t12E9760\n2765\t346DF\t3872C1\n2766\t34710\t1C278C0\n2767\t34743\t707EA1\n2768\t34774\t8C6221\n2769\t347A7\t1DC7260\n2770\t347D8\t607C61\n2771\t3480B\t1306361\n2772\t3483C\t14C6D61\n2773\t3486F\t5C7B41\n2774\t348A0\t1A47221\n2775\t348D3\t527880\n2776\t34904\tEE7841\n2777\t34937\t1D879C0\n2778\t34968\t828AA1\n2779\t3499B\t1925321\n2780\t349CC\t18E8F60\n2781\t349FF\t5A6FA0\n2782\t34A30\t1C47A61\n2783\t34A63\tD07201\n2784\t34A94\t2E9341\n2785\t34AC7\t1DA7721\n2786\t34AF8\tE05FA1\n2787\t34B2B\t1906A01\n2788\t34B5C\t16E67A1\n2789\t34B8F\t3C6F60\n2790\t34BC0\t1629401\n2791\t34BF3\tB462A1\n2792\t34C24\t8E6641\n2793\t34C57\t15C7220\n2794\t34C88\t462C0\n2795\t34CBB\t1D47600\n2796\t34CEC\t1C866E1\n2797\t34D1F\tDC8B01\n2798\t34D50\t1A272E1\n2799\t34D83\t3078A0\n2800\t34DB4\t2A5BC0\n2801\t34DE7\t1BC7DE1\n2802\t34E18\tA07BE1\n2803\t34E4B\tF07961\n2804\t34E7C\tEC6A40\n2805\t34EAF\tBA8120\n2806\t34EE0\t1027281\n2807\t34F13\t3271C1\n2808\t34F44\tCE66A1\n2809\t34F77\t7A7D20\n2810\t34FA8\t205D00\n2811\t34FDB\t1D08540\n2812\t3500C\t1AE69E1\n2813\t3503F\t3A7741\n2814\t35070\t408A21\n2815\t350A3\tB07F41\n2816\t350D4\t2E6641\n2817\t35107\tFC7400\n2818\t35138\t627F60\n2819\t3516B\t1708800\n2820\t3519C\t6E61A0\n2821\t351CF\t7C7461\n2822\t35200\tA06D61\n2823\t35233\t746341\n2824\t35264\t4C6200\n2825\t35297\tBC6AA1\n2826\t352C8\t207360\n2827\t352FB\t1328221\n2828\t3532C\t10E7640\n2829\t3535F\t367821\n2830\t35390\t606381\n2831\t353C3\t1B67601\n2832\t353F4\tAE8120\n2833\t35427\t548201\n2834\t35458\t471A1\n2835\t3548B\t9668C1\n2836\t354BC\t16859C0\n2837\t354EF\t3079C1\n2838\t35520\tA05D20\n2839\t35553\t1B08C01\n2840\t35584\t2080A0\n2841\t355B7\t9464C0\n2842\t355E8\t407AC0\n2843\t3561B\t1106461\n2844\t3564C\t2073A0\n2845\t3567F\t706CE0\n2846\t356B0\t6056A0\n2847\t356E3\t347B61\n2848\t35714\t206221\n2849\t35747\t508901\n2850\t35778\t7279A1\n2851\t357AB\t205DC0\n2852\t357DC\t2062E1\n2853\t3710D\t206080\n2854\t372E2\t205D60\n2855\t38537\t2067E1\n2856\t39B52\t2064E1\n2857\t3ADF3\t205B60\n2858\t3B73A\t206B21\n2859\t3BAF3\t2E5420\n2860\t3C80A\tE06540\n2861\t3C83D\t474C1\n2862\t3C86E\tA06600\n2863\t3C8A1\t209620\n2864\t3C8D2\t408140\n2865\t3C905\t607741\n2866\t3C936\t206340\n2867\t3CBC3\t2054C0\n2868\t3D50A\t207F21\n2869\t3F5DF\t606300\n2870\t3F628\t207461\n2871\t3F65B\t208081\n2872\t3F95E\t406481\n2873\t3FC4F\t2086A0\n2874\t3FC80\t207660\n2875\t3FD79\t2065A1\n2876\t400F8\t206620\n2877\t40187\t2067E1\n2878\t401D4\t207D40\n2879\t40225\t206B60\n2880\t405A4\t205F61\n2881\t406CF\t2063C1\n2882\t407F8\t206961\n2883\t40B79\t206561\n2884\t40CA2\t2073A0\n2885\t40DCF\t2072A1\n2886\t40F86\t205FC1\n2887\t41215\t1D86961\n2888\t41686\t14E6301\n2889\t416B9\t1507A81\n2890\t416EA\t1C66A20\n2891\t4171D\t11C6B01\n2892\t4174E\t4E7640\n2893\t41781\tD07C00\n2894\t417B2\tE09281\n2895\t417E5\t1DA6CE1\n2896\t41816\t16E6220\n2897\t41849\t1306E00\n2898\t4187A\t1C28020\n2899\t418AD\t5C8200\n2900\t418DE\t2C6501\n2901\t41911\t328101\n2902\t41942\t49400\n2903\t41975\t387E20\n2904\t419A6\tCE7021\n2905\t419D9\t1907C00\n2906\t41A0A\t1A45F21\n2907\t41A3D\t5A71C0\n2908\t41A6E\t2E8B00\n2909\t41AA1\t309780\n2910\t41AD2\tA091E0\n2911\t41B05\t387120\n2912\t41B36\t8E5B20\n2913\t41B69\tF075E0\n2914\t41B9A\t1C272A0\n2915\t41BCD\t7C6FE0\n2916\t41BFE\t2A6061\n2917\t41C31\t907520\n2918\t41C62\t20ADA0\n2919\t41C95\tFC6861\n2920\t41CC6\t10E6C21\n2921\t41CF9\t1707A80\n2922\t41D2A\tE08720\n2923\t41D5D\t3A6E80\n2924\t41D8E\t2E7181\n2925\t41DC1\t708820\n2926\t41DF2\t498E1\n2927\t41E25\t1105F60\n2928\t41E56\t6E6760\n2929\t41E89\tD07261\n2930\t41EBA\t609EC1\n2931\t41EED\t1906E00\n2932\t41F1E\tEE6AC0\n2933\t41F51\t307AE0\n2934\t41F82\t208AC0\n2935\t41FB5\tB06F61\n2936\t41FE6\tAE6F20\n2937\t42019\t367540\n2938\t4204A\tE06741\n2939\t4207D\t706661\n2940\t420AE\t4E55E1\n2941\t420E1\t5091A1\n2942\t42112\t46BA0\n2943\t42145\tA09240\n2944\t42176\t206C80\n2945\t421A9\t409221\n2946\t421DA\t46B00\n2947\t4220D\t606CE1\n2948\t4223E\t208621\n2949\t42271\t406361\n2950\t422A2\t205F01\n2951\t422D5\t2068A0\n2952\t423BA\t3883E1\n2953\t4292F\t2E7EE1\n2954\t42960\tF06820\n2955\t42993\t1C26F41\n2956\t429C4\t326980\n2957\t429F7\t4E6600\n2958\t42A28\t1707501\n2959\t42A5B\tE08CA0\n2960\t42A8C\tD06E81\n2961\t42ABF\t4A241\n2962\t42AF0\t1906760\n2963\t42B23\t2E7680\n2964\t42B54\t308800\n2965\t42B87\tA08FA1\n2966\t42BB8\t906F00\n2967\t42BEB\t20AF40\n2968\t42C1C\t7079A0\n2969\t42C4F\tE074E0\n2970\t42C80\t3686A1\n2971\t42CB3\t49EA0\n2972\t42CE4\t306AE1\n2973\t42D17\t608C20\n2974\t42D48\t706E81\n2975\t42D7B\t208240\n2976\t42DAC\t5085A1\n2977\t42DDF\tE061A0\n2978\t42E10\t408A81\n2979\t42E43\t46100\n2980\t42E9E\tE06C20\n2981\t42ED1\t207BA1\n2982\t42F02\t6071C0\n2983\t42F35\t406B81\n2984\t42F66\t2060E0\n2985\t4306D\tA068C1\n2986\t4309E\t606E61\n2987\t430D1\t4065E0\n2988\t43102\t2059A1\n2989\t43237\t207000\n2990\t43282\t206221\n2991\t432CF\tE06A01\n2992\t43320\t208AE1\n2993\t43353\t606201\n2994\t43384\t207000\n2995\t433B7\t406CE0\n2996\t433E8\t46E81\n2997\t4341B\tA07121\n2998\t4344C\t207CA0\n2999\t4347F\t606A60\n3000\t434B0\t4062C0\n3001\t434E3\t207AA0\n3002\t43576\t6074C0\n3003\t435A9\t205F61\n3004\t435DA\t405E21\n3005\t4360D\t2075C0\n3006\t4363E\t206400\n3007\t4369F\t207EC1\n3008\t437CA\t206841\n3009\t438F5\t2063E0\n3010\t43A1E\t606780\n3011\t43AAD\t207A21\n3012\t43ADE\t206F61\n3013\t43B33\t206B00\n3014\t43C74\t308A20\n3015\t43D03\t2E6F81\n3016\t43D34\t706DA0\n3017\t43D67\tE06FC1\n3018\t43D98\t506B40\n3019\t43DCB\t48AC0\n3020\t43DFC\tA08D00\n3021\t43E2F\t20AE41\n3022\t43E60\t4083C0\n3023\t43E93\t608EE1\n3024\t43EC4\tF075A1\n3025\t43EF7\t12E6DC0\n3026\t43F28\tD07681\n3027\t43F5B\t1C46861\n3028\t43F8C\t1506281\n3029\t43FBF\t10E6500\n3030\t43FF0\t3075A1\n3031\t44023\t207861\n3032\t44054\t1706720\n3033\t44087\t2E6C00\n3034\t440B8\t707261\n3035\t440EB\tE059E0\n3036\t4411C\t506F00\n3037\t4414F\t4E6480\n3038\t44180\tA06DA1\n3039\t441B3\t406D81\n3040\t441E4\t207880\n3041\t44265\t206CA1\n3042\t44374\t2068C0\n3043\t44411\t607D41\n3044\t44442\t46301\n3045\t44475\t406980\n3046\t444A6\t206BC0\n3047\t444D9\t206EA0\n3048\t4452C\t207300\n3049\t448AF\tA061C1\n3050\t44994\t46040\n3051\t449C7\t606941\n3052\t449F8\t207240\n3053\t44A2B\t407440\n3054\t44A5C\t306B20\n3055\t44A8F\t2E6A00\n3056\t44AC0\t506381\n3057\t44AF3\t469A1\n3058\t44B24\tA08200\n3059\t44B57\t3074A0\n3060\t44B88\t2E67A1\n3061\t44BBB\t506701\n3062\t44BEC\t208621\n3063\t44C1F\tE067A0\n3064\t44C50\t466C1\n3065\t44C83\t6077C0\n3066\t44CB4\t2067C0\n3067\t44CE7\tA05FC0\n3068\t44D18\t207101\n3069\t44D4B\t406B41\n3070\t44D7C\t207101\n3071\t44DAF\t206EE1\n3072\t44DF6\tA05EE0\n3073\t44FAD\t469A1\n3074\t44FDE\t6060A0\n3075\t45011\t207CC0\n3076\t45042\t406C01\n3077\t45075\t46BC0\n3078\t450CA\t605C00\n3079\t450FD\t208921\n3080\t4512E\t4053C1\n3081\t45161\t208261\n3082\t45192\tA062A1\n3083\t451C5\t6079C1\n3084\t451F6\t206CA1\n3085\t45241\t4053A1\n3086\t45272\t467E1\n3087\t452A5\tE063E0\n3088\t452D6\t207D01\n3089\t45309\t606AA0\n3090\t4533A\t207521\n3091\t4536D\t407840\n3092\t4539E\t307700\n3093\t453D1\t1AE64C1\n3094\t45402\t7078E0\n3095\t45435\t1C26820\n3096\t45466\t507BA0\n3097\t45499\t2E7141\n3098\t454CA\t48140\n3099\t454FD\tE08300\n3100\t4552E\t20A680\n3101\t45561\tA07AA1\n3102\t45592\t608D21\n3103\t455C5\t4084E0\n3104\t455F6\t207401\n3105\t45629\t205F80\n3106\t4584C\t606DA1\n3107\t4587F\t207161\n3108\t458B0\t405200\n3109\t459D9\t2086C0\n3110\t45A0A\t606C21\n3111\t45A3D\t325D21\n3112\t49190\t2E6280\n3113\t491C3\t3064C1\n3114\t491F4\t47A60\n3115\t49227\t707360\n3116\t49258\tE05E00\n3117\t4928B\t209EA0\n3118\t492BC\tA063E1\n3119\t492EF\t1D85C80\n3120\t49320\t14E7440\n3121\t49353\t1306260\n3122\t49384\t1C66A20\n3123\t493B7\t387900\n3124\t493E8\tCE5860\n3125\t4941B\t328DC1\n3126\t4944C\t47C21\n3127\t4947F\t1DC7A20\n3128\t494B0\t18E7CC0\n3129\t494E3\t1B06B40\n3130\t49514\t1C48680\n3131\t49547\t1DA6CC0\n3132\t49578\t2C5A80\n3133\t495AB\tB07B61\n3134\t495DC\tE07DE0\n3135\t4960F\t9C78C0\n3136\t49640\t12E6F80\n3137\t49673\t1B260A1\n3138\t496A4\tE27340\n3139\t496D7\t13C7480\n3140\t49708\t8E6AA0\n3141\t4973B\tD46C21\n3142\t4976C\t826660\n3143\t4979F\t586FC1\n3144\t497D0\t1AE83E0\n3145\t49803\t965C00\n3146\t49834\t12271C1\n3147\t49867\t17C6F00\n3148\t49898\t6C66E1\n3149\t498CB\t309E20\n3150\t498FC\t405821\n3151\t4992F\t7C7AE1\n3152\t49960\t16E7561\n3153\t49993\t19467A1\n3154\t499C4\t1C691A0\n3155\t499F7\t1DC8221\n3156\t49A28\t1686B80\n3157\t49A5B\t347401\n3158\t49A8C\t245880\n3159\t49ABF\t389141\n3160\t49AF0\t18E9260\n3161\t49B23\t1506D00\n3162\t49B54\t1C27620\n3163\t49B87\t1D87500\n3164\t49BB8\t2A6FC1\n3165\t49BEB\tD07C21\n3166\t49C1C\tE074A1\n3167\t49C4F\tBC8240\n3168\t49C80\t12E6E00\n3169\t49CB3\t1D47660\n3170\t49CE4\t1426BE1\n3171\t49D17\t19C6460\n3172\t49D48\t6E6E21\n3173\t49D7B\t5468A0\n3174\t49DAC\t209F61\n3175\t49DDF\t11C7AC1\n3176\t49E10\t1AE6341\n3177\t49E43\t1308521\n3178\t49E74\t1827780\n3179\t49EA7\t15C6221\n3180\t49ED8\t287680\n3181\t49F0B\t3676C1\n3182\t49F3C\tA09F60\n3183\t49F6F\t5C8D60\n3184\t49FA0\t14E6B60\n3185\t49FD3\t1D07361\n3186\t4A004\t1626D61\n3187\t4A037\t1BC6801\n3188\t4A068\tCE84C1\n3189\t4A09B\t3292E1\n3190\t4A0CC\t4A4E1\n3191\t4A0FF\tDC7F81\n3192\t4A130\t2C6F20\n3193\t4A163\t1906FE0\n3194\t4A194\t1A279A1\n3195\t4A1C7\t17C6720\n3196\t4A1F8\tAE74E0\n3197\t4A22B\t9070A1\n3198\t4A25C\t607FE0\n3199\t4A28F\t3A9761\n3200\t4A2C0\t6A55C0\n3201\t4A2F3\t1B47280\n3202\t4A324\t10275C1\n3203\t4A357\t1DA7080\n3204\t4A388\t10E80C1\n3205\t4A3BB\t526CE0\n3206\t4A3EC\t2064A0\n3207\t4A41F\t5A8221\n3208\t4A450\t2E7221\n3209\t4A483\tB67341\n3210\t4A4B4\t1C46861\n3211\t4A4E7\t9C6180\n3212\t4A518\t4E7B60\n3213\t4A54B\t308200\n3214\t4A57C\t626A61\n3215\t4A5AF\tFC8FC1\n3216\t4A5E0\tEE5AA0\n3217\t4A613\t1707A01\n3218\t4A644\t1A48061\n3219\t4A677\t726801\n3220\t4A6A8\t8E7980\n3221\t4A6DB\t1106D40\n3222\t4A70C\t4269A0\n3223\t4A73F\tB08921\n3224\t4A770\t1B66660\n3225\t4A7A3\t7094A0\n3226\t4A7D4\tF06BC1\n3227\t4A807\t507EE1\n3228\t4A838\t1B09B61\n3229\t4A86B\t605DC1\n3230\t4A89C\tD073C0\n3231\t4A8CF\t2081A1\n3232\t4A900\t206160\n3233\t4BC8F\t2E5420\n3234\t4C6BA\t5071C0\n3235\t4C6ED\tE06BE1\n3236\t4C71E\t46141\n3237\t4C751\tA07FA1\n3238\t4C782\t208660\n3239\t4C7B5\t407000\n3240\t4C7E6\t207AA0\n3241\t4C819\t606E01\n3242\t4C84A\t2075C0\n3243\t4C87D\t205BE1\n3244\t4CCA2\t205A61\n3245\t4CEED\t205B60\n3246\t4CF6C\t305D80\n3247\t4D03B\t1AE4D41\n3248\t4D06C\t1D06DC1\n3249\t4D09F\tE06160\n3250\t4D0D0\t707660\n3251\t4D103\t2E7281\n3252\t4D134\t305EC1\n3253\t4D167\t47280\n3254\t4D198\t505780\n3255\t4D1CB\tA07380\n3256\t4D1FC\t2099E0\n3257\t4D22F\t407720\n3258\t4D260\t6080C1\n3259\t4D293\t206400\n3260\t4D5A4\t206421\n3261\t4E6CD\t207B80\n3262\t4E7DE\tE05B41\n3263\t4E915\t472A1\n3264\t4E946\tA066A0\n3265\t4E979\t207BE0\n3266\t4E9AA\t4075E1\n3267\t4E9DD\t607520\n3268\t4EA0E\t206DC0\n3269\t4EA41\t205E81\n3270\t4EB54\tE05F61\n3271\t4EC95\t47CC0\n3272\t4ECC6\tA06A00\n3273\t4ECF9\t207BC1\n3274\t4ED2A\t406800\n3275\t4ED5D\t606C81\n3276\t4ED8E\t206380\n3277\t4EDC1\t1D07080\n3278\t4EEEA\tA06780\n3279\t4EF1D\t47321\n3280\t4EF4E\t606960\n3281\t4EF81\t206DA0\n3282\t4EFB2\t207AC0\n3283\t4F13F\t206340\n3284\t4F18A\t405D81\n3285\t4F409\t2080C0\n3286\t4F43A\t606341\n3287\t4F46D\t2071C1\n3288\t4F4BE\t606201\n3289\t4F4F1\t207461\n3290\t4F522\t406400\n3291\t4F555\t46A20\n3292\t4F5B2\tE06B60\n3293\t4F5E5\t208F41\n3294\t4F616\tA06381\n3295\t4F649\t209901\n3296\t4F67A\t607121\n3297\t4F6AD\t406F61\n3298\t4F6DE\t206D41\n3299\t4F95D\t2067A0\n3300\t4F9A8\tA05321\n3301\t4FAE5\t207F00\n3302\t4FB16\t606C21\n3303\t4FB49\t405680\n3304\t4FB7A\t46D60\n3305\t4FE53\tA06C60\n3306\t4FE84\t306B40\n3307\t4FEB7\t1AE6621\n3308\t4FEE8\t1D07040\n3309\t4FF1B\t1C26321\n3310\t4FF4C\t706C01\n3311\t4FF7F\t2E6F60\n3312\t4FFB0\tD069C1\n3313\t4FFE3\t2077C1\n3314\t50014\t5066C0\n3315\t50047\tE07420\n3316\t50078\t47780\n3317\t500AB\t606F21\n3318\t500DC\t2072C1\n3319\t5010F\tA06820\n3320\t50140\t406C01\n3321\t50173\t1D07C61\n3322\t501A4\t18E67E1\n3323\t501D7\t1DC6F21\n3324\t50208\t1C27281\n3325\t5023B\tD06421\n3326\t5026C\t10E60E1\n3327\t5029F\tF06BC1\n3328\t502D0\t480E1\n3329\t50303\t306A41\n3330\t50334\t12E5821\n3331\t50367\t386821\n3332\t50398\t1C45AE1\n3333\t503CB\t1D26C80\n3334\t503FC\t2E67C1\n3335\t5042F\t1DC7320\n3336\t50460\tE077A1\n3337\t50493\t326F61\n3338\t504C4\t1AE76C1\n3339\t504F7\t3C7AC1\n3340\t50528\t1C66D81\n3341\t5055B\t15069C1\n3342\t5058C\t6E69C1\n3343\t505BF\t1D876A0\n3344\t505F0\t20A501\n3345\t50623\t906720\n3346\t50654\t16E6101\n3347\t50687\t386901\n3348\t506B8\t1A46AE1\n3349\t506EB\t1D671C0\n3350\t5071C\t2A6BE1\n3351\t5074F\t1DA73A1\n3352\t50780\tA079A1\n3353\t507B3\t5263E0\n3354\t507E4\t18E6E60\n3355\t50817\t5A6E61\n3356\t50848\t1C249A1\n3357\t5087B\t1327361\n3358\t508AC\tCE6A80\n3359\t508DF\t1586D01\n3360\t50910\t446FC0\n3361\t50943\t567E00\n3362\t50974\t12A6500\n3363\t509A7\tB87C20\n3364\t509D8\t1A67021\n3365\t50A0B\t1B29020\n3366\t50A3C\tAC72A0\n3367\t50A6F\t15C81A1\n3368\t50AA0\tC24600\n3369\t50AD3\tB27481\n3370\t50B04\t12E6D81\n3371\t50B37\tBA7840\n3372\t50B68\t1227321\n3373\t50B9B\t1967641\n3374\t50BCC\tAE5DE1\n3375\t50BFF\t987761\n3376\t50C30\tA27341\n3377\t50C63\t1128060\n3378\t50C94\t14A64E0\n3379\t50CC7\tD87BA0\n3380\t50CF8\t1265101\n3381\t50D2B\t15270A1\n3382\t50D5C\t4C6D00\n3383\t50D8F\t17A77E1\n3384\t50DC0\t607100\n3385\t50DF3\t3470A0\n3386\t50E24\t10A64A0\n3387\t50E57\tFA6CA0\n3388\t50E88\t1828060\n3389\t50EBB\t966A21\n3390\t50EEC\t1686E40\n3391\t50F1F\t1B88180\n3392\t50F50\t48C60\n3393\t50F83\tF46F80\n3394\t50FB4\t18C6E61\n3395\t50FE7\t586680\n3396\t51018\tE26BE0\n3397\t5104B\t1D46DE1\n3398\t5107C\t288B41\n3399\t510AF\t15A6BE1\n3400\t510E0\tE0A961\n3401\t51113\t925F20\n3402\t51144\t14E7560\n3403\t51177\tDA7740\n3404\t511A8\t1847A81\n3405\t511DB\t1766E80\n3406\t5120C\t487C40\n3407\t5123F\t13C7461\n3408\t51270\t2679A0\n3409\t512A3\tB07120\n3410\t512D4\t18A7CA1\n3411\t51307\t388E40\n3412\t51338\t1C692A0\n3413\t5136B\t1546761\n3414\t5139C\t8A6760\n3415\t513CF\t1BA6C00\n3416\t51400\t867240\n3417\t51433\t545D60\n3418\t51464\t1AE7E81\n3419\t51497\t7A7420\n3420\t514C8\t1C26401\n3421\t514FB\t1366601\n3422\t5152C\t1486741\n3423\t5155F\t1786901\n3424\t51590\t2474E1\n3425\t515C3\t367E00\n3426\t515F4\t1AA69E0\n3427\t51627\t1187A00\n3428\t51658\t1646CC0\n3429\t5168B\t1726B00\n3430\t516BC\t6C6801\n3431\t516EF\t19A8C41\n3432\t51720\tE09901\n3433\t51753\tF27280\n3434\t51784\t16E9021\n3435\t517B7\t5C8661\n3436\t517E8\t1A27EA0\n3437\t5181B\t1B68700\n3438\t5184C\t886381\n3439\t5187F\t787400\n3440\t518B0\t826440\n3441\t518E3\tD07DE0\n3442\t51914\t16A69C1\n3443\t51947\t11A6F81\n3444\t51978\t10276E0\n3445\t519AB\t1927A61\n3446\t519DC\t2C64A0\n3447\t51A0F\t1DC8DA0\n3448\t51A40\t4671A1\n3449\t51A73\t328261\n3450\t51AA4\t10853C0\n3451\t51AD7\t9A75C1\n3452\t51B08\t1C469C0\n3453\t51B3B\tB683E1\n3454\t51B6C\tEE5DC1\n3455\t51B9F\t1987B81\n3456\t51BD0\t474C1\n3457\t51C03\tF66701\n3458\t51C34\t14C7A01\n3459\t51C67\t11C84A0\n3460\t51C98\t16269E1\n3461\t51CCB\t1D28161\n3462\t51CFC\t2E7F20\n3463\t51D2F\t1D88DC1\n3464\t51D60\tE07AC0\n3465\t51D93\tD27221\n3466\t51DC4\t16E65E1\n3467\t51DF7\t3CA101\n3468\t51E28\t1C27281\n3469\t51E5B\t1508EC1\n3470\t51E8C\t6E8B80\n3471\t51EBF\t1BC8141\n3472\t51EF0\tA46C61\n3473\t51F23\t9094A1\n3474\t51F54\t16C72C1\n3475\t51F87\tFC6D80\n3476\t51FB8\t14278E0\n3477\t51FEB\t1D68881\n3478\t5201C\t2A8541\n3479\t5204F\t17C7BA0\n3480\t52080\tA0D1C0\n3481\t520B3\tD47D41\n3482\t520E4\t1A86B01\n3483\t52117\t7C7401\n3484\t52148\t1A480C1\n3485\t5217B\t1306B81\n3486\t521AC\t10E8340\n3487\t521DF\t1DC72E1\n3488\t52210\t626D00\n3489\t52243\t706800\n3490\t52274\t10C6481\n3491\t522A7\t387041\n3492\t522D8\t1C27441\n3493\t5230B\t1B46E21\n3494\t5233C\t6A7121\n3495\t5236F\t19C7C21\n3496\t523A0\tE06760\n3497\t523D3\t7478C0\n3498\t52404\t1AE6E20\n3499\t52437\tDC75C0\n3500\t52468\t1C26B61\n3501\t5249B\t19078E0\n3502\t524CC\t8E6EE0\n3503\t524FF\t1DC6C21\n3504\t52530\t208600\n3505\t52563\t7672C1\n3506\t52594\t18EA301\n3507\t525C7\t3C7C20\n3508\t525F8\t606E01\n3509\t5262B\t1946D80\n3510\t5265C\t2E7901\n3511\t5268F\t1DA9401\n3512\t526C0\t48DC1\n3513\t526F3\t326760\n3514\t52724\t1AE6D80\n3515\t52757\tBC7420\n3516\t52788\tE07101\n3517\t527BB\t1108221\n3518\t527EC\tEE6341\n3519\t5281F\t1D874A1\n3520\t52850\t1C66DA0\n3521\t52883\t3074E1\n3522\t528B4\t18E5C20\n3523\t528E7\t387921\n3524\t52918\t20A141\n3525\t5294B\t1D07FC1\n3526\t5297C\t2E7A61\n3527\t529AF\t1DC6600\n3528\t529E0\t1C27040\n3529\t52A13\tB472E1\n3530\t52A44\t1AE6B61\n3531\t52A77\t3A70C1\n3532\t52AA8\tA07D21\n3533\t52ADB\t1706461\n3534\t52B0C\t4E6D40\n3535\t52B3F\t9C7AA1\n3536\t52B70\t427520\n3537\t52BA3\t906E80\n3538\t52BD4\t18E6380\n3539\t52C07\t3C7C01\n3540\t52C38\tE07DC1\n3541\t52C6B\t1D06AE1\n3542\t52C9C\t2E6C21\n3543\t52CCF\t5A7F20\n3544\t52D00\t209BE1\n3545\t52D33\t727100\n3546\t52D64\t10E69A0\n3547\t52D97\tF07441\n3548\t52DC8\t406E00\n3549\t52DFB\t506600\n3550\t52E2C\t46BC0\n3551\t52E5F\t1B06A21\n3552\t52E90\t606B80\n3553\t52EC3\t947180\n3554\t52EF4\t1AE60A0\n3555\t52F27\t1D06701\n3556\t52F58\t206200\n3557\t52F8B\t13C7300\n3558\t52FBC\t4C6160\n3559\t52FEF\tD07B61\n3560\t53020\tE26BC1\n3561\t53053\t5869C1\n3562\t53084\t12A6420\n3563\t530B7\t1308261\n3564\t530E8\tE06961\n3565\t5311B\t15C7AA0\n3566\t5314C\tAE8AA0\n3567\t5317F\t3486E1\n3568\t531B0\t1226A61\n3569\t531E3\tBA6901\n3570\t53214\t12E7761\n3571\t53247\t1D483A0\n3572\t53278\t626B60\n3573\t532AB\t15866E1\n3574\t532DC\tAC7260\n3575\t5330F\t3069C0\n3576\t53340\t1C68381\n3577\t53373\t3881C1\n3578\t533A4\t16A6A80\n3579\t533D7\t15082E0\n3580\t53408\tA07961\n3581\t5343B\t1BA6EE0\n3582\t5346C\tCE7B61\n3583\t5349F\tB26581\n3584\t534D0\t1827521\n3585\t53503\tDC6561\n3586\t53534\t1A87BA0\n3587\t53567\t1527781\n3588\t53598\tA26421\n3589\t535CB\t9869C1\n3590\t535FC\t8A6F01\n3591\t5362F\tB093A1\n3592\t53660\t1427EA1\n3593\t53693\t11C8680\n3594\t536C4\t1AA7220\n3595\t536F7\t967B81\n3596\t53728\tE06BA0\n3597\t5375B\t15A6001\n3598\t5378C\t6E8740\n3599\t537BF\t528A21\n3600\t537F0\t1246A40\n3601\t53823\t3CA1C1\n3602\t53854\t14E8420\n3603\t53887\t1B27360\n3604\t538B8\t476C0\n3605\t538EB\t1B86EC0\n3606\t5391C\t287361\n3607\t5394F\t567841\n3608\t53980\t1628160\n3609\t539B3\t7A60A1\n3610\t539E4\t18A5B20\n3611\t53A17\t19673E1\n3612\t53A48\t466A20\n3613\t53A7B\t1DCA2E0\n3614\t53AAC\tEE9021\n3615\t53ADF\tD26981\n3616\t53B10\t1A269C0\n3617\t53B43\t5C8AC1\n3618\t53B74\t1C86DC1\n3619\t53BA7\t1D68620\n3620\t53BD8\t267981\n3621\t53C0B\t787121\n3622\t53C3C\t2C6501\n3623\t53C6F\t767820\n3624\t53CA0\t10278C0\n3625\t53CD3\t9A7320\n3626\t53D04\t14A5C41\n3627\t53D37\tB67480\n3628\t53D68\tE05181\n3629\t53D9B\t19A76A0\n3630\t53DCC\t8E7D41\n3631\t53DFF\t327240\n3632\t53E30\t1C28FA1\n3633\t53E63\t7C7EC1\n3634\t53E94\t16E8501\n3635\t53EC7\t1D28C00\n3636\t53EF8\t246D20\n3637\t53F2B\t1786FA1\n3638\t53F5C\t6C60A0\n3639\t53F8F\t307421\n3640\t53FC0\t1A487C0\n3641\t53FF3\tFC83C1\n3642\t54024\t10C6141\n3643\t54057\t1707CC1\n3644\t54088\tA05A60\n3645\t540BB\t1BC71A0\n3646\t540EC\t10E9041\n3647\t5411F\t746840\n3648\t54150\t1C46F41\n3649\t54183\t3A68C1\n3650\t541B4\t18E9481\n3651\t541E7\t1927001\n3652\t54218\t826A81\n3653\t5424B\t1986801\n3654\t5427C\t2A7F60\n3655\t542AF\t908121\n3656\t542E0\tE06DE1\n3657\t54313\t9C7C80\n3658\t54344\t16C6A01\n3659\t54377\t11084C0\n3660\t543A8\t47761\n3661\t543DB\t1D87600\n3662\t5440C\t4EA541\n3663\t5443F\t547280\n3664\t54470\t607DE1\n3665\t544A3\tBC7120\n3666\t544D4\t1AE9E61\n3667\t54507\t1726DA0\n3668\t54538\t20EEA1\n3669\t5456B\t19C8600\n3670\t5459C\t2E6921\n3671\t545CF\t3686A1\n3672\t54600\tE07280\n3673\t54633\t5A8961\n3674\t54664\t4270E0\n3675\t54697\t1B674E1\n3676\t546C8\tA07B81\n3677\t546FB\t17C7741\n3678\t5472C\t207740\n3679\t5475F\tD48061\n3680\t54790\t4077C1\n3681\t547C3\t1DA8B41\n3682\t547F4\t469A1\n3683\t54827\t1D0A021\n3684\t54858\t207480\n3685\t5488B\tD07AE1\n3686\t548BC\t44E01\n3687\t548EF\tF07A01\n3688\t54920\t405841\n3689\t54953\t726DE0\n3690\t54984\t2080C0\n3691\t549B7\t1D471C1\n3692\t549E8\t306500\n3693\t54A1B\t1909001\n3694\t54A4C\t706121\n3695\t54A7F\t607441\n3696\t54AB0\t1946FC0\n3697\t54AE3\t465A1\n3698\t54B14\t505F41\n3699\t54B47\tA06861\n3700\t54B78\t1B091A1\n3701\t54BAB\t2080E1\n3702\t54BDC\t1B469A1\n3703\t54C0F\t18E68E1\n3704\t54C40\t385760\n3705\t54C73\t1C26681\n3706\t54CA4\t906360\n3707\t54CD7\t4E70A1\n3708\t54D08\t3C7061\n3709\t54D3B\tE07600\n3710\t54D6C\t1D066A0\n3711\t54D9F\t1AE65C0\n3712\t54DD0\t307281\n3713\t54E03\t49AA1\n3714\t54E34\t1D46E21\n3715\t54E67\t2E7260\n3716\t54E98\t7060E0\n3717\t54ECB\t406181\n3718\t54EFC\t1D47960\n3719\t54F2F\t208AA0\n3720\t54F60\t5072E1\n3721\t54F93\tE06800\n3722\t54FC4\t477C1\n3723\t54FF7\t1D48E01\n3724\t55028\tA07D00\n3725\t5505B\t1D47041\n3726\t5508C\t207861\n3727\t550BF\t1DC74A0\n3728\t550F0\t18E7AC0\n3729\t55123\t327840\n3730\t55154\t1A26541\n3731\t55187\t7C5980\n3732\t551B8\t4E6E01\n3733\t551EB\tF07301\n3734\t5521C\tE09121\n3735\t5524F\t1DA6B40\n3736\t55280\t1C861A1\n3737\t552B3\tD062A0\n3738\t552E4\t1C26FC0\n3739\t55317\t3C7380\n3740\t55348\t2E8141\n3741\t5537B\t1D07040\n3742\t553AC\t47880\n3743\t553DF\t3079C1\n3744\t55410\t1AE6DE0\n3745\t55443\t1706B80\n3746\t55474\t6091E0\n3747\t554A7\t906A81\n3748\t554D8\t4E78A0\n3749\t5550B\t3877E0\n3750\t5553C\t1C26BC1\n3751\t5556F\t1B26AE0\n3752\t555A0\t16E7721\n3753\t555D3\t326FC1\n3754\t55604\t20C601\n3755\t55637\tF06FE1\n3756\t55668\t2E7980\n3757\t5569B\t708341\n3758\t556CC\tE06640\n3759\t556FF\t1D084E1\n3760\t55730\t18E8021\n3761\t55763\tD07280\n3762\t55794\t46EA0\n3763\t557C7\t1906181\n3764\t557F8\t1AE6E01\n3765\t5582B\t307520\n3766\t5585C\tA08841\n3767\t5588F\t3C7141\n3768\t558C0\t20B6C0\n3769\t558F3\t1D26961\n3770\t55924\tE06D00\n3771\t55957\tD05C61\n3772\t55988\tCE7581\n3773\t559BB\t13C7521\n3774\t559EC\t1C679A0\n3775\t55A1F\t1307021\n3776\t55A50\tEC69C1\n3777\t55A83\t11C5FE1\n3778\t55AB4\t47CA0\n3779\t55AE7\t527140\n3780\t55B18\t2C7161\n3781\t55B4B\t1D869E0\n3782\t55B7C\t1626C21\n3783\t55BAF\t1D67F40\n3784\t55BE0\t18E7081\n3785\t55C13\tBC7060\n3786\t55C44\t408960\n3787\t55C77\t366C21\n3788\t55CA8\tAE7A60\n3789\t55CDB\t1DC70A1\n3790\t55D0C\t1C27141\n3791\t55D3F\t1507641\n3792\t55D70\t14E5BA0\n3793\t55DA3\t387660\n3794\t55DD4\t20B740\n3795\t55E07\t347E61\n3796\t55E38\t2E7C01\n3797\t55E6B\t1BC6180\n3798\t55E9C\tE07701\n3799\t55ECF\t1B26C01\n3800\t55F00\t1C87B60\n3801\t55F33\t5C85C1\n3802\t55F64\t488A1\n3803\t55F97\tB07461\n3804\t55FC8\tEE5CC0\n3805\t55FFB\t1DA6B61\n3806\t5602C\tA07501\n3807\t5605F\t967F01\n3808\t56090\t12E7E40\n3809\t560C3\tFC69C0\n3810\t560F4\t206800\n3811\t56127\t326AC1\n3812\t56158\t2E63C0\n3813\t5618B\t3C98E0\n3814\t561BC\tE07261\n3815\t561EF\t1D06A21\n3816\t56220\t18E65A1\n3817\t56253\t5A6820\n3818\t56284\t48381\n3819\t562B7\t3089E0\n3820\t562E8\t6E75C0\n3821\t5631B\t3A7241\n3822\t5634C\t60A261\n3823\t5637F\t1B07DE1\n3824\t563B0\t16E7BA0\n3825\t563E3\tD095C1\n3826\t56414\t206881\n3827\t56447\t1D48B80\n3828\t56478\t10E9041\n3829\t564AB\t708500\n3830\t564DC\tA06E20\n3831\t5650F\tF06BC1\n3832\t56540\t1AE7340\n3833\t56573\t3C6DC1\n3834\t565A4\t47420\n3835\t565D7\t908320\n3836\t56608\t2E70C1\n3837\t5663B\t1D65FA0\n3838\t5666C\tE068E1\n3839\t5669F\t306D20\n3840\t566D0\t8E7E60\n3841\t56703\t1707561\n3842\t56734\t207041\n3843\t56767\tD071A1\n3844\t56798\t4E7221\n3845\t567CB\t1B28060\n3846\t567FC\t408EA1\n3847\t5682F\t5071A0\n3848\t56860\t46940\n3849\t56893\t1107020\n3850\t568C4\tA06861\n3851\t568F7\t706281\n3852\t56928\t207101\n3853\t5695B\t1D07821\n3854\t5698C\t608F20\n3855\t569BF\t1907DE0\n3856\t569F0\t1D28A00\n3857\t56A23\t1B075A1\n3858\t56A54\t1D66CE1\n3859\t56A87\t1B28500\n3860\t56AB8\t1D06CA0\n3861\t56AEB\t1D47A81\n3862\t56B1C\t1D661E0\n3863\t56B4F\t1B265C1\n3864\t56B80\t1D26061\n3865\t56BB3\t1D072C0\n3866\t56BE4\t47500\n3867\t56C17\t1B27981\n3868\t56C48\tE062E1\n3869\t56C7B\t1D67FC1\n3870\t56CAC\t207E61\n3871\t56CDF\t1D47E80\n3872\t56D10\tA066A0\n3873\t56D43\t1D09321\n3874\t56D74\t407440\n3875\t56DA7\t1B26AC1\n3876\t56DD8\t205421\n3877\t56E0B\t1D68821\n3878\t56E3C\t606A81\n3879\t56E6F\t1D295A1\n3880\t56EA0\t206E21\n3881\t56ED3\t1D085C1\n3882\t56F04\t1B27FA0\n3883\t56F37\t1D690E1\n3884\t56F68\t1D46340\n3885\t56F9B\t206B00\n3886\t56FCC\t1D07A61\n3887\t56FFF\t1B28041\n3888\t57030\t1D68700\n3889\t57063\t1D298E1\n3890\t57094\t1D06F21\n3891\t570C7\t18E7CC0\n3892\t570F8\t1DC6EA1\n3893\t5712B\t1C664E1\n3894\t5715C\t3479E1\n3895\t5718F\t2E7D60\n3896\t571C0\t387220\n3897\t571F3\tE09020\n3898\t57224\tF06681\n3899\t57257\t1AE6F41\n3900\t57288\t3A74C0\n3901\t572BB\t1C26C00\n3902\t572EC\t906EE0\n3903\t5731F\t10E66A0\n3904\t57350\t3C7A80\n3905\t57383\t49BC0\n3906\t573B4\t1B286E1\n3907\t573E7\t4E6880\n3908\t57418\t327BA1\n3909\t5744B\tA08540\n3910\t5747C\t1507AA0\n3911\t574AF\t20B4C1\n3912\t574E0\t307D21\n3913\t57513\t409141\n3914\t57544\t1D67D21\n3915\t57577\t46881\n3916\t575A8\t5088C0\n3917\t575DB\t608B81\n3918\t5760C\t3C64E0\n3919\t5763F\t207581\n3920\t57670\t1B06E80\n3921\t576A3\t406460\n3922\t576D4\t707E61\n3923\t57707\t1D468E1\n3924\t57738\t46DE1\n3925\t5776B\t3C6AC0\n3926\t5779C\t606A81\n3927\t577CF\t1705AA0\n3928\t57800\t208C21\n3929\t57833\t1D0ABA1\n3930\t57864\t406E81\n3931\t57897\t1B2B861\n3932\t578C8\t1D67C01\n3933\t578FB\t206EA0\n3934\t5792C\t3C7680\n3935\t5795F\t406961\n3936\t57990\tD05F80\n3937\t579C3\t1D26C40\n3938\t579F4\t1D08141\n3939\t57A27\t18E6A20\n3940\t57A58\t3A64A1\n3941\t57A8B\t491A0\n3942\t57ABC\t3267A0\n3943\t57AEF\t2E6EA1\n3944\t57B20\t3C87E1\n3945\t57B53\tE07180\n3946\t57B84\tF05FA0\n3947\t57BB7\t1AE6F41\n3948\t57BE8\t3C8380\n3949\t57C1B\t20A961\n3950\t57C4C\t3069E1\n3951\t57C7F\tA07160\n3952\t57CB0\t3C77E1\n3953\t57CE3\t47161\n3954\t57D14\t1B2C080\n3955\t57D47\t6094A1\n3956\t57D78\tD076A0\n3957\t57DAB\t205F20\n3958\t57DDC\t3C61E0\n3959\t57E0F\t408660\n3960\t57E40\t1D6A6E1\n3961\t57E73\t47081\n3962\t57EA4\t3C76A1\n3963\t57ED7\t2E6A81\n3964\t57F08\t506A81\n3965\t57F3B\tE06E00\n3966\t57F6C\t3C76C1\n3967\t57F9F\t1AE55E1\n3968\t57FD0\t1D478C1\n3969\t58003\t208FA0\n3970\t58034\t3C75A1\n3971\t58067\t2E65E1\n3972\t58098\tD06EC0\n3973\t580CB\tA06D01\n3974\t580FC\t3C7D41\n3975\t5812F\t47EC1\n3976\t58160\t1D09B61\n3977\t58193\tE07220\n3978\t581C4\t3C7D60\n3979\t581F7\t16E6180\n3980\t58228\t307361\n3981\t5825B\t1C26C81\n3982\t5828C\t3C7520\n3983\t582BF\t2E7DE1\n3984\t582F0\t1907500\n3985\t58323\t206961\n3986\t58354\t17C6480\n3987\t58387\t18E6D21\n3988\t583B8\t346F40\n3989\t583EB\t1C67381\n3990\t5841C\t387480\n3991\t5844F\tCE6680\n3992\t58480\t1B301C1\n3993\t584B3\t606F60\n3994\t584E4\t1DA77E1\n3995\t58517\t14E7060\n3996\t58548\tB06DA0\n3997\t5857B\t1C46801\n3998\t585AC\t3CC0A0\n3999\t585DF\t2C6EE1\n4000\t58610\t1306640\n4001\t58643\t47600\n4002\t58674\t1D87AC0\n4003\t586A7\t1C86521\n4004\t586D8\t327D80\n4005\t5870B\t1C274E1\n4006\t5873C\t3CC621\n4007\t5876F\tAE6781\n4008\t587A0\t1D6A7C1\n4009\t587D3\tE06C40\n4010\t58804\t1DC81E1\n4011\t58837\t16E6C41\n4012\t58868\t707480\n4013\t5889B\t206F61\n4014\t588CC\t3C9DC1\n4015\t588FF\t2E85E0\n4016\t58930\t1507B40\n4017\t58963\tA07D41\n4018\t58994\t3C6A41\n4019\t589C7\t18E59C1\n4020\t589F8\tD066A1\n4021\t58A2B\t406B81\n4022\t58A5C\t3CAD40\n4023\t58A8F\tEE6BC1\n4024\t58AC0\t1D26EC0\n4025\t58AF3\t6069C0\n4026\t58B24\t3C7CC1\n4027\t58B57\t1AE65A0\n4028\t58B88\t3091A1\n4029\t58BBB\t6E6F61\n4030\t58BEC\t3C81C0\n4031\t58C1F\t10E71C0\n4032\t58C50\t1106F00\n4033\t58C83\t8E7260\n4034\t58CB4\t3C9E40\n4035\t58CE7\t4E75A1\n4036\t58D18\t907441\n4037\t58D4B\t3C72A0\n4038\t58D7C\t1D09BE0\n4039\t58DAF\t3C7A61\n4040\t58DE0\t365C21\n4041\t58E13\t3C9D20\n4042\t58E44\t1B07080\n4043\t58E77\t3C7460\n4044\t58EA8\t506EC1\n4045\t58EDB\t3C6F41\n4046\t58F0C\t1D44E20\n4047\t58F3F\t3C7580\n4048\t58F70\tD065A1\n4049\t58FA3\t3C9981\n4050\t58FD4\tF06C60\n4051\t59007\t3C8481\n4052\t59038\t2064C0\n4053\t5906B\t1D07FE0\n4054\t5909C\tE06601\n4055\t590CF\t3C9A21\n4056\t59100\t207981\n4057\t59133\t1706EA1\n4058\t59164\t406741\n4059\t59197\t3C7AA1\n4060\t591C8\t606960\n4061\t591FB\t3C8920\n4062\t5922C\t3C6C60\n4063\t5925F\t206B60\n4064\t59290\t3CB0C1\n4065\t592C3\t606900\n4066\t592F4\t3CA641\n4067\t59327\t3CC240\n4068\t59360\t3C73E0\n4069\t59393\t3C9BA1\n4070\t593C4\t474A1\n4071\t593F7\t1D067E0\n4072\t59428\tE07060\n4073\t5945B\t3CD700\n4074\t5948C\t209601\n4075\t594BF\t3C7E81\n4076\t594F0\tA063C0\n4077\t59523\t3CACA0\n4078\t59554\t406421\n4079\t59587\t3C9F60\n4080\t595B8\t607C61\n4081\t595EB\t3C64E0\n4082\t5961C\t206BE1\n4083\t5964F\t3CBE21\n4084\t59680\t3C6F41\n4085\t596B9\t3CD741\n4086\t596EA\t206A40\n4087\t5971D\t3CDC80\n4088\t5974E\tA06300\n4089\t59781\t3CE5A1\n4090\t597B2\t207BE0\n4091\t597E5\t3C82A0\n4092\t59816\t406221\n4093\t59849\t3C8821\n4094\t5987A\t45700\n4095\t598AD\t1D06321\n4096\t598DE\t606C00\n4097\t59911\t3CC0E1\n4098\t59942\t208081\n4099\t59975\t3C9921\n4100\t599A6\tE06061\n4101\t599D9\t3CD181\n4102\t59A0A\t46860\n4103\t59A3D\t307260\n4104\t59A6E\t3F69A0\n4105\t59AA1\t3CC021\n4106\t59AD2\t1C36381\n4107\t59B05\t1D065A0\n4108\t59B36\tB06081\n4109\t59B69\t3CEB21\n4110\t59B9A\t307AC0\n4111\t59BCD\t707F00\n4112\t59BFE\t13F7060\n4113\t59C31\t1DC6F60\n4114\t59C62\t1C36B40\n4115\t59C95\t1186EA1\n4116\t59CC6\t10F7460\n4117\t59CF9\t386BC0\n4118\t59D2A\tF080C0\n4119\t59D5D\t3B7B80\n4120\t59D8E\t18F6260\n4121\t59DC1\t1D86A61\n4122\t59DF2\t1C47080\n4123\t59E25\t1D47861\n4124\t59E56\t3F7980\n4125\t59E89\t3CAC21\n4126\t59EBA\t475C0\n4127\t59EED\tB06741\n4128\t59F1E\t13F5DC0\n4129\t59F51\t1DC7561\n4130\t59F82\t1C36F41\n4131\t59FB5\t19861A0\n4132\t59FE6\tBF6781\n4133\t5A019\t3CC1C1\n4134\t5A04A\t406E00\n4135\t5A07D\t335FC1\n4136\t5A0AE\t1C86CC0\n4137\t5A0E1\t3D0D41\n4138\t5A112\t30A721\n4139\t5A145\t1D88640\n4140\t5A176\t3F7561\n4141\t5A1A9\t3072E1\n4142\t5A1DA\tF06E21\n4143\t5A20D\t1307021\n4144\t5A23E\t18F6C01\n4145\t5A271\tD07EE0\n4146\t5A2A2\t475E1\n4147\t5A2D5\t1D45EC0\n4148\t5A306\tFF6C00\n4149\t5A339\t3F6A21\n4150\t5A36A\tB08781\n4151\t5A39D\t1587300\n4152\t5A3CE\t1BF7340\n4153\t5A401\t906480\n4154\t5A432\t309001\n4155\t5A465\tF86EC1\n4156\t5A496\t4F69C0\n4157\t5A4C9\t3876E0\n4158\t5A4FA\t706B40\n4159\t5A52D\t1B88221\n4160\t5A55E\t10F6B20\n4161\t5A591\t7870C0\n4162\t5A5C2\t3060A1\n4163\t5A5F5\t1186CC0\n4164\t5A626\t4068E1\n4165\t5A659\t507BE1\n4166\t5A68A\t307220\n4167\t5A6BD\t17068E0\n4168\t5A6EE\t705820\n4169\t5A721\tD86D60\n4170\t5A752\t406D21\n4171\t5A785\t3088C1\n4172\t5A7B6\t1DC6D01\n4173\t5A7E9\t13F6C01\n4174\t5A81A\t1D75260\n4175\t5A84D\tB06C00\n4176\t5A87E\t3D9160\n4177\t5A8B1\t3F80A1\n4178\t5A8E2\t336800\n4179\t5A915\t46040\n4180\t5A946\tF86F21\n4181\t5A979\t18F6540\n4182\t5A9AA\t3D3620\n4183\t5A9DD\t707D41\n4184\t5AA0E\t787201\n4185\t5AA41\t10F7361\n4186\t5AA72\t1D87320\n4187\t5AAA5\t306A40\n4188\t5AAD6\tB06CE0\n4189\t5AB09\t1BF5D61\n4190\t5AB3A\t1B074E1\n4191\t5AB6D\t406BC0\n4192\t5AB9E\t507D60\n4193\t5ABD1\t1705E01\n4194\t5AC02\tD87C00\n4195\t5AC35\t986240\n4196\t5AC66\t467C0\n4197\t5ACB5\t1D86521\n4198\t5ACE6\tF06620\n4199\t5AD19\t586740\n4200\t5AD4A\t308280\n4201\t5AD7D\tD07201\n4202\t5ADAE\tB06401\n4203\t5ADE1\t308360\n4204\t5AE12\t7076E0\n4205\t5AE45\t47161\n4206\t5AE76\t1D70680\n4207\t5AEA9\t3F7121\n4208\t5AEDA\t1DC6D20\n4209\t5AF0D\t1C36A81\n4210\t5AF3E\t3B5D00\n4211\t5AF71\t18F6721\n4212\t5AFA2\t1D06FE1\n4213\t5AFD5\tF06F01\n4214\t5B006\t387441\n4215\t5B039\t1BF6521\n4216\t5B06A\tD86881\n4217\t5B09D\t307681\n4218\t5B0CE\t506EA1\n4219\t5B101\tB077E1\n4220\t5B132\t47300\n4221\t5B165\t4071A1\n4222\t5B196\t305DA0\n4223\t5B1C9\t706D40\n4224\t5B1FA\t3864A0\n4225\t5B36B\t8F7061\n4226\t5B39C\t1386C80\n4227\t5B3CF\t1C36C81\n4228\t5B400\t1D870A0\n4229\t5B433\t14F6B00\n4230\t5B464\t5B68C0\n4231\t5B497\t48E01\n4232\t5B4C8\tFC70E0\n4233\t5B4FB\t3C6181\n4234\t5B52C\t1D73A40\n4235\t5B55F\tF089E1\n4236\t5B590\t1DB7781\n4237\t5B5C3\t18F76C0\n4238\t5B5F4\tB875C0\n4239\t5B627\t30A800\n4240\t5B658\t3B73A1\n4241\t5B68B\tCF7480\n4242\t5B6BC\t19879A0\n4243\t5B6EF\tB09341\n4244\t5B720\t1DC76A1\n4245\t5B753\t17F6C81\n4246\t5B784\t3C74C1\n4247\t5B7B7\t46A80\n4248\t5B7E8\t5B7001\n4249\t5B81B\t3F7A20\n4250\t5B84C\t1D09480\n4251\t5B87F\tF06DC0\n4252\t5B8B0\t389B40\n4253\t5B8E3\t1BF8281\n4254\t5B914\t1187620\n4255\t5B947\t307C81\n4256\t5B978\t3B8081\n4257\t5B9AB\t7F6C20\n4258\t5B9DC\t1D71D61\n4259\t5BA0F\t1C36D20\n4260\t5BA40\t1DC66C0\n4261\t5BA73\t17F6941\n4262\t5BAA4\t986EA1\n4263\t5BAD7\t409340\n4264\t5BB08\t15072E0\n4265\t5BB3B\t3F79A1\n4266\t5BB6C\t3B65C1\n4267\t5BB9F\t48A60\n4268\t5BBD0\t1D07301\n4269\t5BC03\t18F7820\n4270\t5BC34\t788541\n4271\t5BC67\tF086A0\n4272\t5BC98\tF068C1\n4273\t5BCCB\tFF75C1\n4274\t5BCFC\t307BC0\n4275\t5BD2F\t30AA61\n4276\t5BD60\t1D7FE61\n4277\t5BD93\t1BF6D20\n4278\t5BDC4\t3F7121\n4279\t5BDF7\tB08580\n4280\t5BE28\t1B87B60\n4281\t5BE5B\tBF6AE0\n4282\t5BE8C\t5871C0\n4283\t5BEBF\t3075C0\n4284\t5BEF0\t1DFC4E0\n4285\t5BF23\t4F71E1\n4286\t5BF54\tD06441\n4287\t5BF87\t709EE0\n4288\t5BFB8\t17069A0\n4289\t5BFEB\t46C80\n4290\t5C01C\t1D7ECA1\n4291\t5C04F\t407D20\n4292\t5C080\t308201\n4293\t5C0B3\t385F00\n4294\t5C0E4\t1BF5CA0\n4295\t5C117\t1BB4540\n4296\t5C148\tF06E41\n4297\t5C17B\t786DA0\n4298\t5C1AC\t3F6A41\n4299\t5C1DF\t1D06C41\n4300\t5C210\t47521\n4301\t5C243\t506E01\n4302\t5C274\tB06DA1\n4303\t5C2A7\t1D382E1\n4304\t5C2D8\t30A1E1\n4305\t5C30B\t1D70B41\n4306\t5C33C\t708680\n4307\t5C36F\t408500\n4308\t5C3A0\t1D7DB21\n4309\t5C3D3\t3077A1\n4310\t5C404\t1DFC600\n4311\t5C449\t13F66C1\n4312\t5C47A\t3862A0\n4313\t5C4AD\t1C37520\n4314\t5C4DE\t3B7180\n4315\t5C511\t3F6D40\n4316\t5C542\tF865C0\n4317\t5C575\tF07D80\n4318\t5C5A6\t905E61\n4319\t5C5D9\t18F73C0\n4320\t5C60A\t1D07400\n4321\t5C63D\t48D61\n4322\t5C66E\t387F40\n4323\t5C6A1\t1BF6941\n4324\t5C6D2\t1B86D20\n4325\t5C705\tB07881\n4326\t5C736\tD88660\n4327\t5C769\t30A6C1\n4328\t5C79A\t1D7F7C1\n4329\t5C7CD\t708BE1\n4330\t5C7FE\t787E40\n4331\t5C831\t45721\n4332\t5C862\t1706C41\n4333\t5C895\t408600\n4334\t5C8C6\t377B00\n4335\t5C8F9\t3098C0\n4336\t5C92A\t1D7D980\n4337\t5C95D\t586840\n4338\t5C98E\t1D7BF61\n4339\t5C9C1\t1D7C560\n4340\t5CA2E\t1D7D241\n4341\t5CACB\t1D7DEE1\n4342\t5CB06\t3F6220\n4343\t5CB39\tD86BA0\n4344\t5CB6A\tF06800\n4345\t5CB9D\tF06CA0\n4346\t5CBCE\t467E1\n4347\t5CC01\t786380\n4348\t5CC32\tB06CC0\n4349\t5CC65\t1BB1520\n4350\t5CC96\t308600\n4351\t5CCC9\t1D07080\n4352\t5CCFA\t707260\n4353\t5CD2D\t1D7F3E1\n4354\t5CD5E\t407280\n4355\t5CD91\t1DFACA0\n4356\t5CDC2\t307801\n4357\t5CDF5\t1D7A201\n4358\t5CE26\t706780\n4359\t5CE59\t1D7C000\n4360\t5CE8A\t307820\n4361\t5CEBD\t406BA0\n4362\t5CEEE\t1D77DA0\n4363\t5CF21\t1DFB9C1\n4364\t5CF74\t307B01\n4365\t5D003\t1BB0E40\n4366\t5D034\t307AC0\n4367\t5D067\t1D7C8C1\n4368\t5D098\t1B3D321\n4369\t5D0CB\t1D77640\n4370\t5D104\t1D7ADC1\n4371\t5D137\t1BBCBA0\n4372\t5D168\t1DF9740\n4373\t5D19B\t1DFA900\n4374\t5D1D4\t705F41\n4375\t5D207\tD077C1\n4376\t5D238\t306760\n4377\t5D26B\t1BB0B40\n4378\t5D29C\t1D7B980\n4379\t5D2CF\t306DC0\n4380\t5D300\t1DFB520\n4381\t5D333\t1D78481\n4382\t5D368\t14F6D60\n4383\t5D39B\t13C6F61\n4384\t5D3CC\t1C76C40\n4385\t5D3FF\t347B01\n4386\t5D430\tCF71E0\n4387\t5D463\t7C6FA1\n4388\t5D494\tF0A040\n4389\t5D4C7\t1987861\n4390\t5D4F8\t18F6E00\n4391\t5D52B\t15C7981\n4392\t5D55C\t1B474A0\n4393\t5D58F\t389F41\n4394\t5D5C0\t3B66C1\n4395\t5D5F3\t11C6780\n4396\t5D624\t736460\n4397\t5D657\t1DC74C1\n4398\t5D688\t13F7FA0\n4399\t5D6BB\t1BC6E61\n4400\t5D6EC\t1836FE0\n4401\t5D71F\t3B8581\n4402\t5D750\t8F7BA0\n4403\t5D783\tBC6E60\n4404\t5D7B4\tB09E40\n4405\t5D7E7\t1386A20\n4406\t5D818\t1C87E21\n4407\t5D84B\t1D876C0\n4408\t5D87C\t1337300\n4409\t5D8AF\tB07AE1\n4410\t5D8E0\t386B01\n4411\t5D913\t3874A1\n4412\t5D944\t30CD41\n4413\t5D977\t1D084A0\n4414\t5D9A8\t17F8B41\n4415\t5D9DB\t1DC7800\n4416\t5DA0C\t1C37540\n4417\t5DA3F\t3F6C21\n4418\t5DA70\t10F83E0\n4419\t5DAA3\t5C7901\n4420\t5DAD4\tF06D21\n4421\t5DB07\t15082E0\n4422\t5DB38\t1BF9300\n4423\t5DB6B\t17C6461\n4424\t5DB9C\t1737061\n4425\t5DBCF\tD087C1\n4426\t5DC00\t3C6EA0\n4427\t5DC33\tFC70C1\n4428\t5DC64\t4AB00\n4429\t5DC97\t1BB24A0\n4430\t5DCC8\t7F7CC0\n4431\t5DCFB\t1DB6981\n4432\t5DD2C\t1B363A0\n4433\t5DD5F\t789620\n4434\t5DD90\t3F8C01\n4435\t5DDC3\t3B8320\n4436\t5DDF4\t40A9C1\n4437\t5DE27\t1187AA1\n4438\t5DE58\tFF5F60\n4439\t5DE8B\t5B7C20\n4440\t5DEBC\t1C462E0\n4441\t5DEEF\t9097A1\n4442\t5DF20\t3F65A0\n4443\t5DF53\t1D7C381\n4444\t5DF84\t305DC0\n4445\t5DFB7\t307380\n4446\t5DFE8\tBF7681\n4447\t5E01B\t1B89E01\n4448\t5E04C\t70B3A1\n4449\t5E07F\t509641\n4450\t5E0B0\t4F63E1\n4451\t5E0E3\t1D31EA0\n4452\t5E114\t46A40\n4453\t5E147\tBF7461\n4454\t5E178\t407000\n4455\t5E1AB\t1D785A1\n4456\t5E1DC\t1786DC1\n4457\t5E20F\t1BBBA00\n4458\t5E240\tF886E0\n4459\t5E273\t1DF7AC1\n4460\t5E2A4\t1D3B7A1\n4461\t5E2D7\t1BB9121\n4462\t5E308\t1D76A21\n4463\t5E33B\t1D3B2C1\n4464\t5E36C\t1D76BE0\n4465\t5E39F\t1B39181\n4466\t5E3D0\t1D78540\n4467\t5E403\t1DB9160\n4468\t5E434\t1BB7CE1\n4469\t5E467\t1D78EC0\n4470\t5E498\t1DBC6C1\n4471\t5E4CB\t1BB6BE1\n4472\t5E4FC\t1D78A01\n4473\t5E52F\t1D3DEC1\n4474\t5E560\t1BB7E80\n4475\t5E593\t1D78920\n4476\t5E5C4\t1D3D4C1\n4477\t5E5F7\t1BB6C40\n4478\t5E628\t1D78800\n4479\t5E65B\t1D3E101\n4480\t5E68C\t1BB7A81\n4481\t5E6BF\t1D76DC1\n4482\t5E6F0\t1DBAB60\n4483\t5E723\t1B365A1\n4484\t5E754\t1D778A0\n4485\t5E787\t1D396A1\n4486\t5E7B8\t3082A1\n4487\t5E7EB\t1DF69C0\n4488\t5E81C\t706D61\n4489\t5E84F\t1B36EE1\n4490\t5E880\t407201\n4491\t5E8B3\t1D76E40\n4492\t5E8E4\t1D3D880\n4493\t5E917\t1D75D01\n4494\t5E948\t1B377C1\n4495\t5E97B\t1D387A1\n4496\t5E9AC\t1BB97E1\n4497\t5E9DF\t1D39040\n4498\t5EA10\t3066A1\n4499\t5EA43\t1D76E20\n4500\t5EA74\t1B36741\n4501\t5EAA7\t1DBC1E1\n4502\t5EAD8\t1D76AE1\n4503\t5EB0B\t1B37401\n4504\t5EB3C\t306AE0\n4505\t5EB6F\t1D36181\n4506\t5EBA0\t1BB7D01\n4507\t5EBD3\t1D36B81\n4508\t5EC04\t1BB7280\n4509\t5EC37\t1D37280\n4510\t5EC68\t1BB6540\n4511\t5EC9B\t1D38DE0\n4512\t5ECCC\t1BB6A01\n4513\t5ECFF\t306DA0\n4514\t5ED30\t1D76DE0\n4515\t5ED63\t1D37F21\n4516\t5ED94\t406F01\n4517\t5EDC7\t1BB9F61\n4518\t5EDF8\t45FC1\n4519\t5EE2B\t1D3AEC0\n4520\t5EE5C\t307941\n4521\t5EE8F\t1BB6E60\n4522\t5EEC0\t306BA0\n4523\t5EEF3\t1DBA1E1\n4524\t5EF24\t1B37060\n4525\t5EF57\t306200\n4526\t5EF88\t1D768C1\n4527\t5EFBB\t1DB91E1\n4528\t5EFEC\t1B39800\n4529\t5F01F\t1D39D81\n4530\t5F050\t1BB6D00\n4531\t5F083\tB072E1\n4532\t5F0B4\t1D76FC0\n4533\t5F0E7\t47500\n4534\t5F118\t1D376A0\n4535\t5F14B\tF06DC0\n4536\t5F17C\t1BBA0E0\n4537\t5F1AF\t309181\n4538\t5F1E0\t1DB71E0\n4539\t5F213\t7078A0\n4540\t5F244\t306581\n4541\t5F277\t18F6FC1\n4542\t5F2A8\t1D06641\n4543\t5F2DB\t1C36DA1\n4544\t5F30C\t787280\n4545\t5F33F\t3F6A81\n4546\t5F370\t1BB6F01\n4547\t5F3A3\t46A01\n4548\t5F3D4\t586DE0\n4549\t5F407\t1BF6B01\n4550\t5F438\t1D76E40\n4551\t5F46B\t1C36FA0\n4552\t5F49C\t3068C1\n4553\t5F4CF\t3F6341\n4554\t5F500\t1DB7E80\n4555\t5F533\tF075A0\n4556\t5F564\t507661\n4557\t5F597\t1BF5E80\n4558\t5F5C8\t1D86BA1\n4559\t5F5FB\t30A320\n4560\t5F62C\t1BB5EE1\n4561\t5F65F\tB06E80\n4562\t5F690\t1D77040\n4563\t5F6C3\t47FA0\n4564\t5F6F4\t1DB80E1\n4565\t5F727\t406760\n4566\t5F758\t1B372C1\n4567\t5F78B\t3F62E0\n4568\t5F7BC\t586D61\n4569\t5F7EF\t308C60\n4570\t5F820\t1DC66A0\n4571\t5F853\t13F6D41\n4572\t5F884\t1B06641\n4573\t5F8B7\tF06721\n4574\t5F8E8\t3873A0\n4575\t5F91B\t10F6581\n4576\t5F94C\t3B7621\n4577\t5F97F\t1C365C0\n4578\t5F9B0\t1DC7020\n4579\t5F9E3\t18F6CA1\n4580\t5FA14\t1D06C81\n4581\t5FA47\t47E20\n4582\t5FA78\tD08180\n4583\t5FAAB\t3F7460\n4584\t5FADC\tF88020\n4585\t5FB0F\t1C74EA1\n4586\t5FB40\t5C6EA1\n4587\t5FB73\t17F6E40\n4588\t5FBA4\t3B7EE0\n4589\t5FBD7\tB074E1\n4590\t5FC08\t1D86A80\n4591\t5FC3B\t8F72E1\n4592\t5FC6C\t1D371C1\n4593\t5FC9F\t1C367A1\n4594\t5FCD0\t387CC0\n4595\t5FD03\t1C86240\n4596\t5FD34\t388640\n4597\t5FD67\t3083A0\n4598\t5FD98\t1DB6120\n4599\t5FDCB\t3F7AC1\n4600\t5FDFC\t15067C0\n4601\t5FE2F\tF08701\n4602\t5FE60\tFC77A0\n4603\t5FE93\t13F6EC0\n4604\t5FEC4\t3B7341\n4605\t5FEF7\t1C35740\n4606\t5FF28\t1D86D41\n4607\t5FF5B\tCF6920\n4608\t5FF8C\t1D76981\n4609\t5FFBF\t49520\n4610\t5FFF0\t3B6240\n4611\t60023\t18F7BA1\n4612\t60054\tB87201\n4613\t60087\t707F20\n4614\t600B8\t1DC7841\n4615\t600EB\t3F7221\n4616\t6011C\t1386A20\n4617\t6014F\t30A760\n4618\t60180\t705CE0\n4619\t601B3\t1BF7881\n4620\t601E4\t1B366E0\n4621\t60217\tF07AA0\n4622\t60248\tD889C0\n4623\t6027B\t7F6D81\n4624\t602AC\t1986E81\n4625\t602DF\t47861\n4626\t60310\t385E01\n4627\t60343\t3F73E0\n4628\t60374\t1D072E1\n4629\t603A7\tB08200\n4630\t603D8\t906C21\n4631\t6040B\tFF6581\n4632\t6043C\t1106DA1\n4633\t6046F\t308A60\n4634\t604A0\t3F79E0\n4635\t604D3\tBF7500\n4636\t60504\t1D35F20\n4637\t60537\tF075C0\n4638\t60568\tD05F20\n4639\t6059B\t10F75C1\n4640\t605CC\t17075A1\n4641\t605FF\t462E1\n4642\t60630\t387C01\n4643\t60663\t1BF5F21\n4644\t60694\t1D36F01\n4645\t606C7\t4082C1\n4646\t606F8\t786160\n4647\t6072B\t3F6021\n4648\t6075C\tF08241\n4649\t6078F\t307261\n4650\t607C0\t588E21\n4651\t607F3\t4F5A21\n4652\t60824\t3D3AA1\n4653\t60857\tB06941\n4654\t60888\t1B86C00\n4655\t608BB\t46B00\n4656\t608EC\t507FC1\n4657\t6091F\tF06320\n4658\t60950\t1D07580\n4659\t60983\t306340\n4660\t609B4\t3D2B61\n4661\t609E7\t706C60\n4662\t60A18\t387380\n4663\t60A4B\t47021\n4664\t60A7C\t3D0580\n4665\t60AAF\tB06D20\n4666\t60AE0\t507400\n4667\t60B13\t3065A1\n4668\t60B44\t408420\n4669\t60B77\t3D33E0\n4670\t60BA8\t706AC0\n4671\t60BDB\t3D0C20\n4672\t60C0C\t305CE0\n4673\t60C3F\t306A01\n4674\t60CA8\t3D3DA0\n4675\t60CDB\t306181\n4676\t60D0C\tF067A0\n4677\t60D3F\t3D03A1\n4678\t60D70\t46561\n4679\t60DA3\t3CBDA0\n4680\t60DD4\t407021\n4681\t60E07\t3CE2C0\n4682\t60E38\t308EE0\n4683\t60E6B\t3D36E0\n4684\t60E9C\t707241\n4685\t60ECF\t3D1560\n4686\t60F00\t406421\n4687\t60F33\t3CF5E1\n4688\t60F9A\tF861E0\n4689\t61029\t3F7881\n4690\t6105A\t3D2F60\n4691\t6108D\t465A1\n4692\t610BE\tD07360\n4693\t610F1\t10F6E80\n4694\t61122\t3CD181\n4695\t61155\tF08DA1\n4696\t61186\t1D05621\n4697\t611B9\t18F6460\n4698\t611EA\t1DC6840\n4699\t6121D\t1C357A1\n4700\t6124E\t388520\n4701\t61281\t3F5FE1\n4702\t612B2\t3CC541\n4703\t612E5\t3084E0\n4704\t61316\t1B85C21\n4705\t61349\t1BF7281\n4706\t6137A\t3D20E1\n4707\t613AD\tB07241\n4708\t613DE\t787981\n4709\t61411\t47740\n4710\t61442\t3CACA0\n4711\t61475\tF07F41\n4712\t614A6\t1D06220\n4713\t614D9\t3F77E1\n4714\t6150A\t3CB620\n4715\t6153D\t1C371C0\n4716\t6156E\t3B73E1\n4717\t615A1\t1BF6261\n4718\t615D2\t3CECA1\n4719\t61605\t307E01\n4720\t61636\t1786021\n4721\t61669\t4F74C0\n4722\t6169A\t3CA861\n4723\t616CD\t1C474C0\n4724\t616FE\t986801\n4725\t61731\t18F6001\n4726\t61762\t3CCC41\n4727\t61795\t707B00\n4728\t617C6\t1D07821\n4729\t617F9\t3F79E0\n4730\t6182A\t3CC381\n4731\t6185D\t1C37481\n4732\t6188E\t3374E0\n4733\t618C1\t1BF66E1\n4734\t618F2\t3CC9C0\n4735\t61925\t47401\n4736\t61956\t1B075C1\n4737\t61989\tFF68A1\n4738\t619BA\t3C79A1\n4739\t619ED\tF085E1\n4740\t61A1E\t386A60\n4741\t61A51\t1BF6BC1\n4742\t61A82\t3CE9A1\n4743\t61AB5\t3087A1\n4744\t61AE6\t1D071E1\n4745\t61B19\t3F6C21\n4746\t61B4A\t1D85CA1\n4747\t61B7D\t1C377A0\n4748\t61BAE\t3B6BC0\n4749\t61BE1\t17F72A0\n4750\t61C12\t386F61\n4751\t61C45\tB07760\n4752\t61C76\t11075E0\n4753\t61CA9\t4F63C0\n4754\t61CDA\t1DC74C0\n4755\t61D0D\t1C378C0\n4756\t61D3E\tD06421\n4757\t61D71\t18F75A0\n4758\t61DA2\t3B6D01\n4759\t61DD5\t469C1\n4760\t61E06\t1D377E0\n4761\t61E39\t3F83A1\n4762\t61E6A\t1D86F20\n4763\t61E9D\tF090A1\n4764\t61ECE\t3B5D21\n4765\t61F01\t13F6AE0\n4766\t61F32\t386B81\n4767\t61F65\t1B36900\n4768\t61F96\t1587660\n4769\t61FC9\tCF5C80\n4770\t61FFA\t1DB6A41\n4771\t6202D\t30AC61\n4772\t6205E\t3F56C0\n4773\t62091\t1BF7B00\n4774\t620C2\t5B6180\n4775\t620F5\t1C37EA0\n4776\t62126\t1DF6941\n4777\t62159\t3C5DE1\n4778\t6218A\t17C6A00\n4779\t621BD\t408101\n4780\t621EE\t3C62E1\n4781\t62221\t14F7900\n4782\t62252\t386340\n4783\t62285\t1C46F60\n4784\t622B6\t1307A81\n4785\t622E9\t8F60E1\n4786\t6231A\t1DC76E0\n4787\t6234D\t49741\n4788\t6237E\tB86E00\n4789\t623B1\t18F92A0\n4790\t623E2\t3C7E21\n4791\t62415\t1C36E80\n4792\t62446\t1D469C1\n4793\t62479\t3859A0\n4794\t624AA\t1D88220\n4795\t624DD\tF09421\n4796\t6250E\t3B7D80\n4797\t62541\t13F6BA0\n4798\t62572\t384F60\n4799\t625A5\t1C46B61\n4800\t625D6\t1907021\n4801\t62609\t10F6A21\n4802\t6263A\t1DC7BA0\n4803\t6266D\t30A4E1\n4804\t6269E\t307DA0\n4805\t626D1\t1BF7C80\n4806\t62702\tFC6A60\n4807\t62735\t1C37520\n4808\t62766\t1D87CE0\n4809\t62799\t3F7C80\n4810\t627CA\t7C79E1\n4811\t627FD\tB08D81\n4812\t6282E\t347180\n4813\t62861\t17F6621\n4814\t62892\t3C6BC1\n4815\t628C5\t47F60\n4816\t628F6\tF87640\n4817\t62929\t7F6AE0\n4818\t6295A\t5C7400\n4819\t6298D\tF04C41\n4820\t629BE\tD07681\n4821\t629F1\t18F82C1\n4822\t62A22\t1D87140\n4823\t62A55\t1B46EC1\n4824\t62A86\t1D36B21\n4825\t62AB9\t3F53C0\n4826\t62AEA\t387A00\n4827\t62B1D\t308240\n4828\t62B4E\t3B8681\n4829\t62B81\t13F7261\n4830\t62BB2\t1DB6120\n4831\t62BE5\t1C466C0\n4832\t62C16\t1705E80\n4833\t62C49\tFF6B40\n4834\t62C7A\t3C8C40\n4835\t62CAD\t7065A0\n4836\t62CDE\t707F21\n4837\t62D11\t1BF6E01\n4838\t62D42\t1D06360\n4839\t62D75\t1C372A0\n4840\t62DA6\t986341\n4841\t62DD9\t3F7601\n4842\t62E0A\t3C89C1\n4843\t62E3D\t463A1\n4844\t62E6E\t1386BC0\n4845\t62EA1\t17F6280\n4846\t62ED2\t3B5BA0\n4847\t62F05\t1C47421\n4848\t62F36\t1D06220\n4849\t62F69\tBF7CE1\n4850\t62F9A\t307760\n4851\t62FCD\tF06760\n4852\t62FFE\t1B86E40\n4853\t63031\t18F6400\n4854\t63062\tD879C0\n4855\t63095\t308EE0\n4856\t630C6\t1185DC1\n4857\t630F9\tCF6DA0\n4858\t6312A\t5067E0\n4859\t6315D\tB07B81\n4860\t6318E\t1507161\n4861\t631C1\t13F70C0\n4862\t631F2\tB05F20\n4863\t63225\t46FE0\n4864\t63256\tF86761\n4865\t63289\t4F8460\n4866\t632BA\t7867C0\n4867\t632ED\t406260\n4868\t6331E\t3F75E0\n4869\t63351\t1BF6480\n4870\t63382\t506CC0\n4871\t633B5\t307621\n4872\t633E6\t10F65E1\n4873\t63419\tB06E01\n4874\t6344A\t8F6440\n4875\t6347D\t3078E0\n4876\t634AE\t7F7600\n4877\t634E1\t7060E1\n4878\t63512\t46B21\n4879\t63545\tB06541\n4880\t63576\t3078C1\n4881\t635A9\t406C80\n4882\t635DA\t306A20\n4883\t63627\t7078A0\n4884\t63658\t1D86620\n4885\t636A7\t14F74C1\n4886\t636D8\t1D06B61\n4887\t6370B\t1C76860\n4888\t6373C\t386E21\n4889\t6376F\t3F7441\n4890\t637A0\t3B7720\n4891\t637D3\t491A0\n4892\t63804\t1DC6880\n4893\t63837\t18F82A1\n4894\t63868\t19856A1\n4895\t6389B\t1C37AC1\n4896\t638CC\t3C7940\n4897\t638FF\t10F64C1\n4898\t63930\t9881A0\n4899\t63963\tF07820\n4900\t63994\t1D06941\n4901\t639C7\t17F7221\n4902\t639F8\t307961\n4903\t63A2B\t30BB80\n4904\t63A5C\t1186BE0\n4905\t63A8F\t3F5FC0\n4906\t63AC0\t788AC0\n4907\t63AF3\tB085C1\n4908\t63B24\t1D06600\n4909\t63B57\t1C86820\n4910\t63B88\tD05D41\n4911\t63BBB\t49741\n4912\t63BEC\t1507581\n4913\t63C1F\tBF63E0\n4914\t63C50\t3876C1\n4915\t63C83\tF06301\n4916\t63CB4\t1B07680\n4917\t63CE7\t1BF77C0\n4918\t63D18\t376B20\n4919\t63D4B\t308960\n4920\t63D7C\t506D20\n4921\t63DAF\t3F68C1\n4922\t63DE0\t409D21\n4923\t63E13\t4F5DE0\n4924\t63E44\t47660\n4925\t63E77\tF05BE1\n4926\t63EA8\t308060\n4927\t63EDB\tB07E60\n4928\t63F0C\t305E00\n4929\t63F3F\t709C21\n4930\t63F70\t3866C1\n4931\t63FFD\t1BF7841\n4932\t6402E\t1D076A1\n4933\t64061\t46A01\n4934\t64092\t3B6A01\n4935\t640C5\t3F6F60\n4936\t640F6\t3878A0\n4937\t64129\tF07D40\n4938\t6415A\t706020\n4939\t6418D\t30A4C0\n4940\t641BE\t506C00\n4941\t641F1\tB07CA1\n4942\t64222\t4098C0\n4943\t64255\t707F40\n4944\t64286\t46E21\n4945\t642B9\tF07081\n4946\t642EA\t3072A1\n4947\t6431D\tB071E1\n4948\t6434E\t306821\n4949\t64381\t406940\n4950\t643B2\t306841\n4951\t644A7\t7074E1\n4952\t644D8\t4073E1\n4953\t6450B\t306800\n4954\t645D0\t706081\n4955\t64661\t307720\n4956\t64692\t7068C1\n4957\t646E1\t307B40\n4958\t64712\t3062A0\n4959\t64745\t705C41\n4960\t64776\t307600\n4961\t647A9\t405BE1\n4962\t64902\t308120\n4963\t64935\t1D06921\n4964\t64966\t1C35AA0\n4965\t64999\t307561\n4966\t649CA\tF060E0\n4967\t649FD\t46FA1\n4968\t64A2E\tB07361\n4969\t64A61\t786521\n4970\t64A92\t1BB6901\n4971\t64AC5\t1335CA0\n4972\t64AF6\t1B764A0\n4973\t64B29\tDC7BA1\n4974\t64B5A\tCF7720\n4975\t64B8D\t9B75E1\n4976\t64BBE\t836120\n4977\t64BF1\t15C73C0\n4978\t64C22\tFC6C01\n4979\t64C55\t17B68C0\n4980\t64C86\t1337720\n4981\t64CB9\t11C65A0\n4982\t64CEA\t8B5AC1\n4983\t64D1D\tB88EC1\n4984\t64D4E\tF0A441\n4985\t64D81\t13C74C1\n4986\t64DB2\t17B77A1\n4987\t64DE5\t1789A00\n4988\t64E16\t1C79881\n4989\t64E49\t7C8081\n4990\t64E7A\t8F7BE1\n4991\t64EAD\t547341\n4992\t64EDE\t345621\n4993\t64F11\t1BB7C20\n4994\t64F42\t18F9760\n4995\t64F75\t1535BE0\n4996\t64FA6\t1838701\n4997\t64FD9\t3894A0\n4998\t6500A\t7B56E1\n4999\t6503D\t577D81\n" -> [w26]
    shift-right: [w21] -> w7
    shift-left: string[] [] -> [w22]
    i -> [w24]
    stop <- w19 stop-if-true
    n2 = Match Pattern(string=w26, regular expression=w25) -> (before substring=w23:string, after substring=w20:string)  [unwired: 1 in, 2 out]
    n3 = Empty String/Path?(string/path=w20) -> (empty?=w19:bool)
    n4 = Insert Into Array(array=w22, index=w24, new element=w23) -> (w21:string[])
  }
  n5 = for {
    tunnel: w7 -> [w41] mode=indexing
    tunnel: [w39] -> w16 mode=indexing
    tunnel: [w38] -> w15 mode=indexing
    tunnel: [w29] -> w14 mode=indexing
    tunnel: [w28] -> w6 mode=indexing
    tunnel: [w27] -> w13 mode=indexing
    w36 = u32 0
    n6 = Scan From String(format string="%d\\t%x\\t%x", input string=w41, default 1=0, default 2=w36, default 3=w36) -> (output 1=w39:i32, output 2=w38:u32, output 3=w29:u32)  [unwired: 2 in, 3 out]
    n7 = Compound Arithmetic op=AND(w29, u32 33423360 ("value")) -> (w30:u32)
    n8 = Compound Arithmetic op=AND(w29, u32 131040 ("value")) -> (w33:u32)
    n9 = Logical Shift(y=-5, x=w33) -> (x << y=w27:u32)
    n10 = Logical Shift(y=-17, x=w30) -> (x << y=w28:u32)
  }
  "Sr No" <- w16
  "Clk Ticks" <- w15
  "Chan+Energy" <- w14
  "Energy" <- w13
  "Channel" <- w6
  n11 = Build Array(w16, w15, w14, w6, w13) -> (w12:u32[][])
  n12 = call <vilib>:"Histogram.vi"("intervals"=255, "X"=w6) -> ("Histogram: h(x)"=w3:i32[], "Histogram Graph"=→"Histogram Graph":T1)  [unwired: 5 in, 3 out]
  n13 = Transpose 2D Array(2D array=w12) -> (transposed array=→"appended array":u32[][])
  n14 = Reshape Array(w3, w4, w4) -> (w2:i32[][])
  "output array" <- w2
  n15 = call-poly <vilib>:"Plot Helper.vi"("z matrix"=w2, "y vector"=w1, "x vector"=w1) -> ("3D Plot lvclass Array out"=→"CZT Count Map":refnum<class "3D Plot Datatype.lvclass">[])  [unwired: 3 in, 5 out]
